vi "Omniax_mDrive_XYZ_MM_BR_RES.vi"() -> ()   [LabVIEW 2009]
uses:
  <vilib>/Instr/_visa.llb/VISA Configure Serial Port (Instr).vi
panel:
  out "Z Backlash steps/sec 2":i32
  out "Z Backlash 2":i32
  out "Z Holding Current % 2":i32
  out "Z Run Current % 2":i32
  out "Z offset mm 2":dbl
  out "Z mm/rev 2":dbl
  out "Z steps/rev 2":u32
  out "Z scan steps/sec MV step/sec 2":i32
  out "Z MINPOS 2":i32=-94296
  out "Z MAXPOS  2":i32=-34296
  out "Z COM PORT 2":refnum<visa-resource-name>="COM5"
  in  "Z Scan set 2":bool
  in  "Z Scan Velocity SP mm/sec 2":dbl
  in  "Z Scan Length SP mm 2":dbl
  in  "Z Move Set 2":bool
  out "Reset Z Motor Steps 2":i32
  in  "Reset Z Position mm 2":dbl
  out "Z Velocity MV mm/sec 2":dbl
  in  "Z Velocity SP mm/sec 2":dbl
  in  "Z Position SP mm 2":dbl
  out "Z Position MV mm 2":dbl
  out "Z Scan velocity MV mm/sec 2":dbl format="%#_6f"
  out "Z Scan length MV mm 2":dbl
  in  "Z Scan Length SP steps 2":i32 min=-460800 max=460800 step=100
  in  "Z Scan OK 2":bool
  in  "Z Velocity SP step/sec 2":i32 min=1 max=102400
  in  "Z Scan Velocity SP steps/sec 2":i32=1 min=1 max=102400 step=1
  in  "Z Go 2":bool
  in  "Z Step SP 2":i32=-20000 min=-460800 max=460800 step=500
  out "Z Position mm PV 2":dbl
  out "R Step PV":i32 max=2000
  out "Z Backlash corr 2":bool
  out "Z in Motion 2":bool
  out "Z Scan 2":bool
  out "Z in Range 2":bool
  out "Y MINPOS 3":i32=-94296
  out "Y MAXPOS 3":i32=-34296
  out "Z COM PORT":refnum<visa-resource-name>="COM5"
  out "Z Backlash steps/sec":i32
  out "Z Backlash":i32
  out "Z Holding Current %":i32
  out "Z Run Current %":i32
  out "Z offset mm":dbl
  out "Z mm/rev":dbl
  out "Z steps/rev":u32
  out "Z scan steps/sec MV step/sec":i32
  out "Z MINPOS":i32=-94296
  out "Z MAXPOS":i32=-34296
  in  "Z Scan set":bool
  in  "Z Scan Velocity SP mm/sec":dbl
  in  "Z Scan Length SP mm":dbl
  in  "Z Move Set":bool
  out "Reset Z Motor Steps":i32
  in  "Reset Z Position mm":dbl
  out "Z Velocity MV mm/sec":dbl
  in  "Z Velocity SP mm/sec":dbl
  in  "Z Position SP mm":dbl
  out "Z Position MV mm":dbl
  out "Z Scan velocity MV mm/sec":dbl format="%#_6f"
  out "Z Scan length MV mm":dbl
  in  "Z Scan Length SP steps":i32 min=-460800 max=460800 step=100
  in  "Z Scan OK":bool
  in  "Z Velocity SP step/sec":i32 min=1 max=102400
  in  "Z Scan Velocity SP steps/sec":i32=1 min=1 max=102400 step=1
  in  "Z Go":bool
  in  "Z Step SP":i32=-20000 min=-460800 max=460800 step=500
  out "Z Position mm PV":dbl
  out "Z Step PV":i32 max=2000
  out "Z Backlash corr":bool
  out "Z in Motion":bool
  out "Z Scan":bool
  out "Z in Range":bool
  out "Reset X Motor Steps":i32
  in  "Reset X Position mm":dbl
  out "X Backlash corr":bool
  out "X  in Motion":bool
  out "X Scan":bool
  out "X  in Range":bool
  out "X Step PV":i32 max=2000
  out "X Position mm PV":dbl
  out "X scan steps/sec MV step/sec":i32
  in  "X Scan set":bool
  in  "X Scan Velocity SP mm/sec":dbl
  in  "X Scan Length SP mm":dbl
  in  "X Move Set":bool
  out "X Velocity MV mm/sec":dbl
  in  "X Velocity SP mm/sec":dbl
  in  "X Position SP mm":dbl
  out "X Position MV mm":dbl
  out "X Scan velocity MV mm/sec":dbl format="%#_6f"
  out "X Scan length MV mm":dbl
  in  "X Scan Length SP steps":i32 min=-460800 max=460800 step=100
  in  "X Scan OK":bool
  in  "X Velocity SP step/sec":i32 min=1 max=102400
  in  "X Scan Velocity SP steps/sec":i32=1 min=1 max=102400 step=1
  in  "X Go":bool
  in  "X Step SP":i32=-20000 min=-460800 max=460800 step=500
  out "X Backlash steps/sec":i32
  out "X Backlash":i32
  out "X Holding Current %":i32
  out "X Run Current %":i32
  out "X offset mm":dbl
  out "X mm/rev":dbl
  out "X steps/rev":u32
  out "X MAXPOS":i32=-34296
  out "X MINPOS":i32=-94296
  out "X COM PORT":refnum<visa-resource-name>="COM5"
  out "Y Backlash corr":bool
  in  "Y Scan set":bool
  in  "Y Scan Velocity SP mm/sec":dbl
  in  "Y Scan Length SP mm":dbl
  in  "Y Move Set":bool
  out "Y Backlash steps/sec":i32
  out "Y Backlash":i32
  out "Y in Motion":bool
  in  "Reset":bool
  out "Reset Y Motor Steps":i32
  in  "Reset Y Position mm":dbl
  out "Y Velocity MV mm/sec":dbl
  in  "Y Velocity SP mm/sec":dbl
  in  "Y Position SP mm":dbl
  out "Y Position MV mm":dbl
  out "Y Holding Current %":i32
  out "Y Run Current %":i32
  out "Y Scan velocity MV mm/sec":dbl format="%#_6f"
  out "Y Scan length MV mm":dbl
  in  "Scan Cancel":bool
  out "Y Position mm PV":dbl
  out "Y offset mm":dbl
  out "Y mm/rev":dbl
  out "Y steps/rev":u32
  out "Y scan steps/sec MV step/sec":i32
  in  "Y Scan Length SP steps":i32 min=-460800 max=460800 step=100
  out "Y Scan":bool
  in  "Y Scan OK":bool
  in  "Scan Go":bool
  in  "Y Velocity SP step/sec":i32 min=1 max=102400
  in  "Y Scan Velocity SP steps/sec":i32=1 min=1 max=102400 step=1
  in  "Stop":bool
  out "Y in Range":bool
  out "Y Step PV":i32 max=2000
  in  "Y Go":bool
  in  "Y Step SP":i32=-20000 min=-460800 max=460800 step=500
  out "Y MINPOS":i32=-94296
  out "Y MAXPOS":i32=-34296
  out "Y COM PORT":refnum<visa-resource-name>="COM5"
  # "LM"
  # "MV"
  # "BL"
  # "SC"
  # "MX"
  # "MY"
  # "MZ"
  # "MR"
types:
  T1 = enum8{"Enabled", "Disabled", "Disabled and Grayed Out"}
  T2 = enum16{"Stop", "Reset", "Run Current", "Holding Current", "Accel Rate", "Decel Rate", "Move to Relative Position", "Move to Absolute Position", "Echo Mode", "Print Parameter", "Send String", "Microstep Resolution", "Set Current Position", "Max Velocity"}
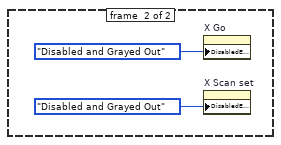
[diagram p2: hidden frame]
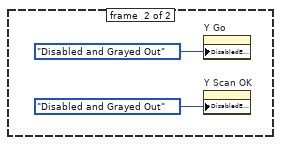
[diagram p5: hidden frame]
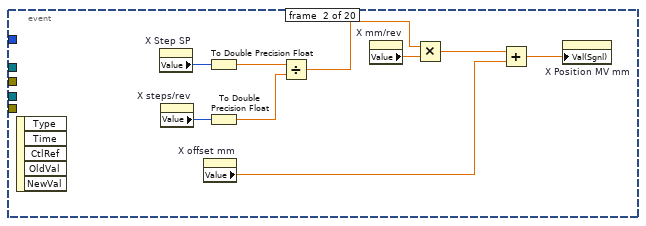
[diagram p8: hidden frame]
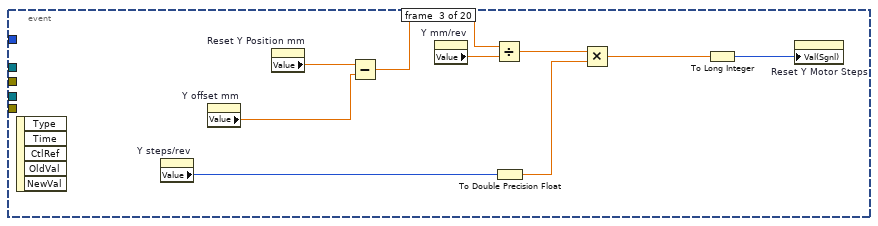
[diagram p9: hidden frame]
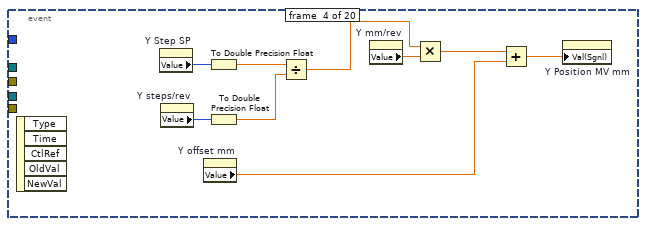
[diagram p10: hidden frame]
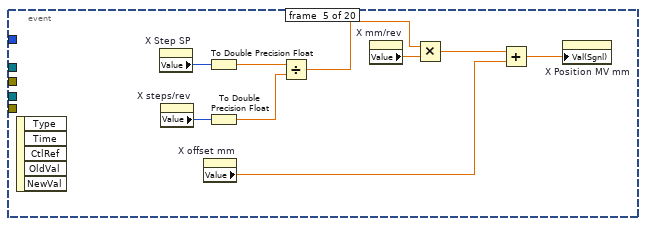
[diagram p11: hidden frame]
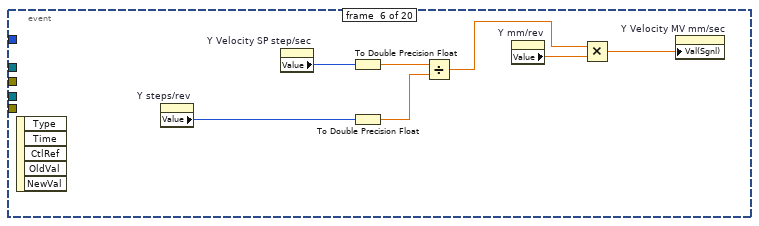
[diagram p12: hidden frame]
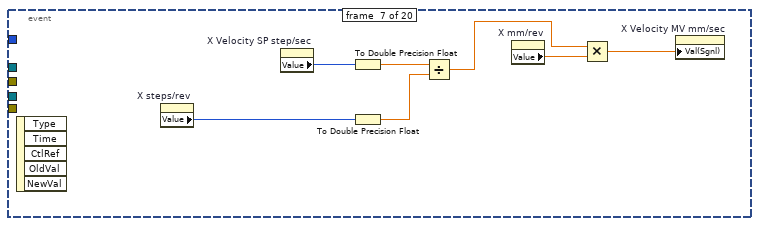
[diagram p13: hidden frame]
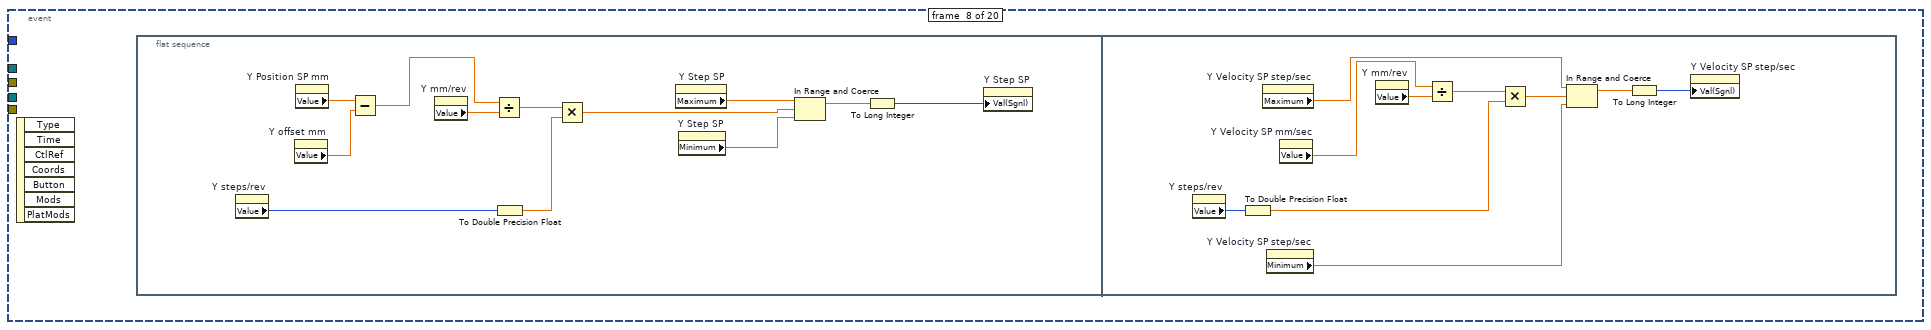
[diagram p14: hidden frame]
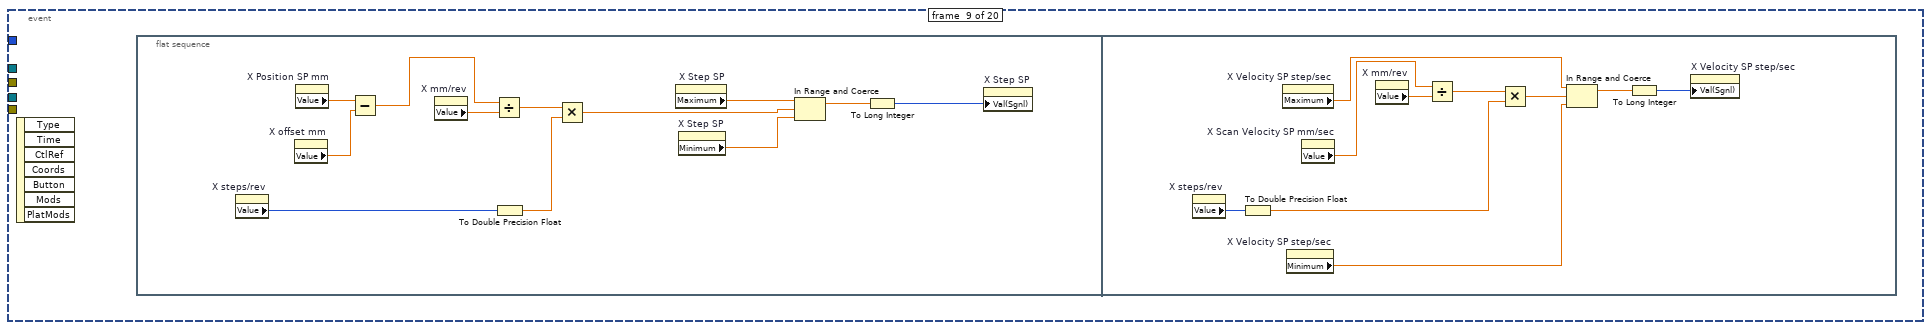
[diagram p15: hidden frame]
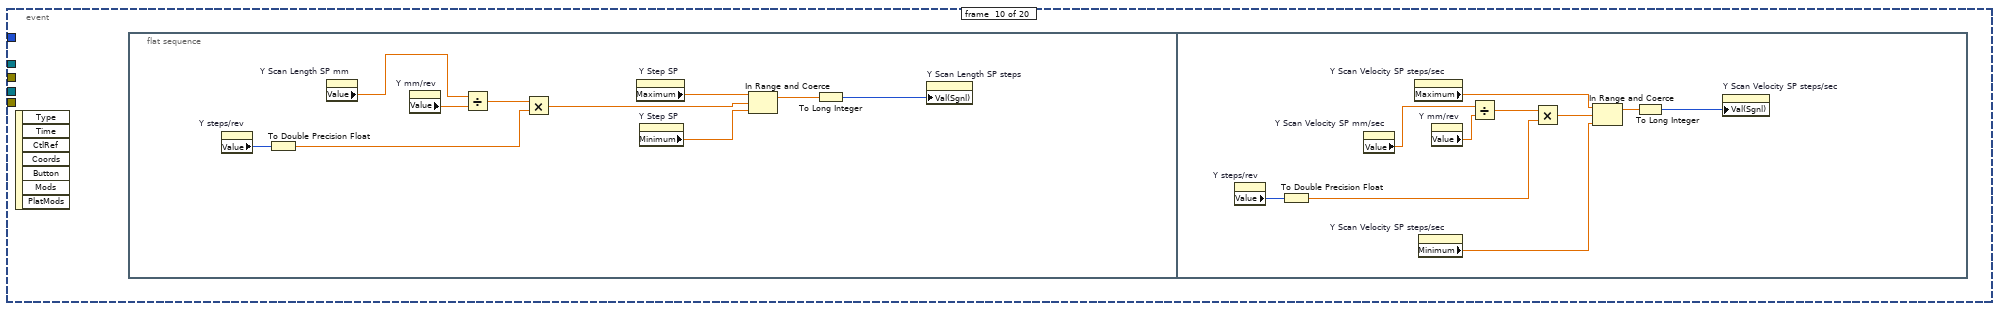
[diagram p16: hidden frame]
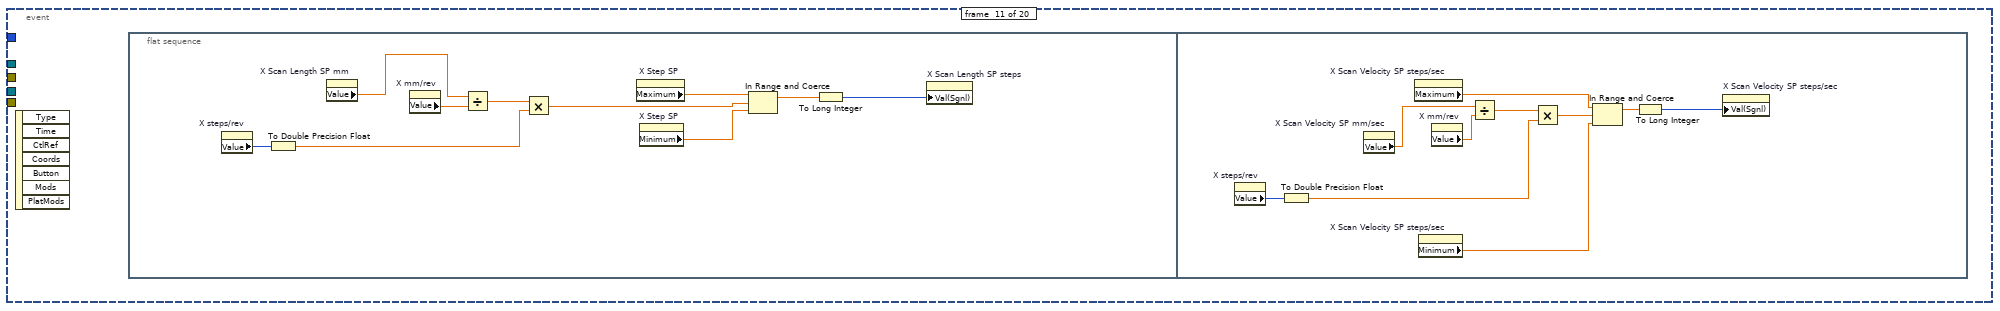
[diagram p17: hidden frame]
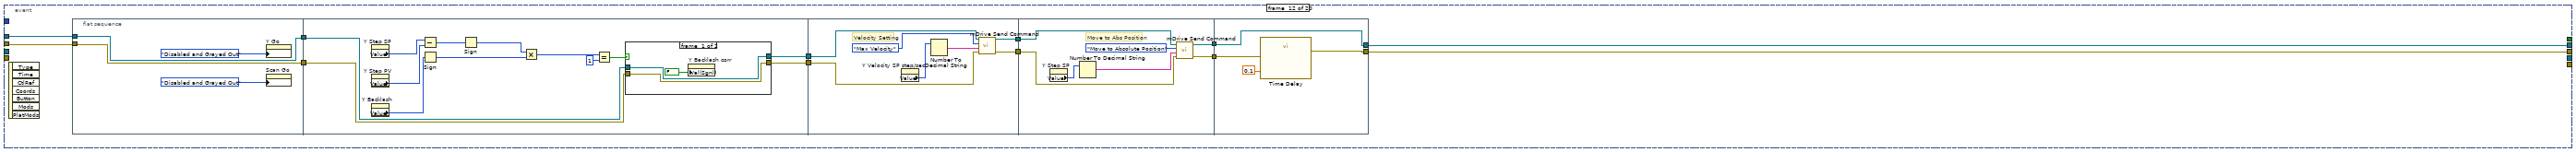
[diagram p18: hidden frame]
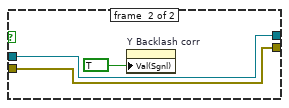
[diagram p19: hidden frame]
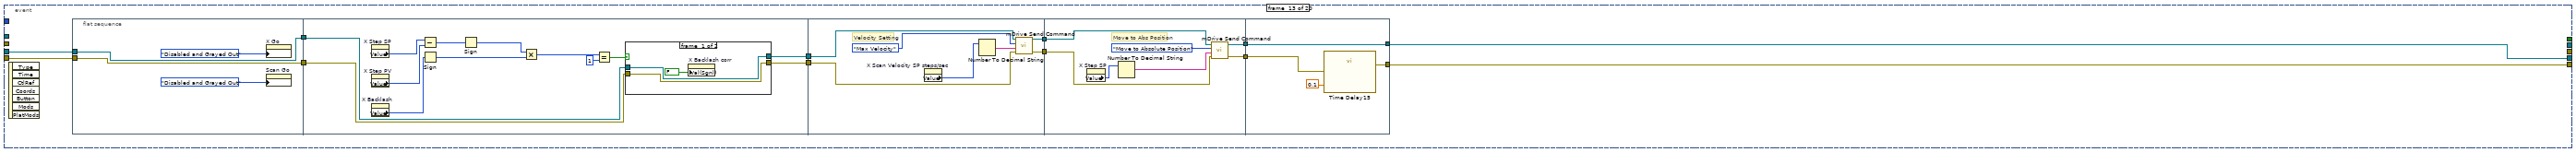
[diagram p20: hidden frame]
diagram:
  w18 = refnum<visa-resource-name> "COM10" ("COM PORT")
  w20 = u16 0 items=["None", "XON/XOFF", "RTS/CTS", "XON/XOFF & RTS/CTS", "DTR/DSR", "XON/XOFF & DTR/DSR"] ("flow control (0:none)")
  w21 = u16 10 items=["1.0"=10, "1.5"=15, "2.0"=20] ("stop bits (10: 1 bit)")
  w31 = refnum<visa-resource-name> "COM8" ("COM PORT")
  w33 = u16 0 items=["None", "XON/XOFF", "RTS/CTS", "XON/XOFF & RTS/CTS", "DTR/DSR", "XON/XOFF & DTR/DSR"] ("flow control (0:none)")
  w34 = u16 10 items=["1.0"=10, "1.5"=15, "2.0"=20] ("stop bits (10: 1 bit)")
  w58 = refnum<visa-resource-name> "COM9" ("COM PORT")
  w60 = u16 0 items=["None", "XON/XOFF", "RTS/CTS", "XON/XOFF & RTS/CTS", "DTR/DSR", "XON/XOFF & DTR/DSR"] ("flow control (0:none)")
  w61 = u16 10 items=["1.0"=10, "1.5"=15, "2.0"=20] ("stop bits (10: 1 bit)")
  # "Stop bits"
  # "Stop bits"
  # "Stop bits"
  n1 = flat-sequence {
    frame #0 {
      "Z Run Current %" <- 60 ("Z Run Current %")
      "Z Holding Current %" <- 25 ("Z Holding Current %")
    }
  }
  n2 = flat-sequence {
    frame #0 {
      w71 = 1.0 ("MM/rev")
      w74 = u32 51200 ("step/rev")
      w69 = 102400 ("Value (Signaling)")
      n3 = property on="X Backlash corr" class="Bool (strict)"("Val(Sgnl)"=FALSE ("Value (Signaling)")) -> ()  [unwired: 2 in, 2 out]
      n4 = property on="X Velocity SP step/sec" class="DigNum (strict)"("Val(Sgnl)"=w69) -> ()  [unwired: 2 in, 2 out]
      n5 = property on="X Scan Velocity SP mm/sec" class="DigNum (strict)"("Val(Sgnl)"=0.1 ("Value (Signaling)")) -> ()  [unwired: 2 in, 2 out]
      n6 = property on="X Scan" class="Bool (strict)"("Val(Sgnl)"=FALSE ("Value (Signaling)")) -> ()  [unwired: 2 in, 2 out]
      n7 = property on="X Velocity SP step/sec" class="DigNum (strict)"("Minimum"=1.0 ("Data Entry Limits:Minimum")) -> ()  [unwired: 2 in, 2 out]
      n8 = To Double Precision Float(number=w74) -> (double precision float=w73:dbl)
      n9 = To Double Precision Float(number=w69) -> (double precision float=w75:dbl)
      n10 = Divide(x=w75, y=w73) -> (x/y=w70:dbl)
      n11 = property on="X Velocity SP step/sec" class="DigNum (strict)"("Maximum"=w75) -> ()  [unwired: 2 in, 2 out]
      n12 = Multiply(x=w70, y=w71) -> (x*y=w72:dbl)
      n13 = property on="X Velocity SP mm/sec" class="DigNum (strict)"("Val(Sgnl)"=w72) -> ()  [unwired: 2 in, 2 out]
      "X Run Current %" <- 60 ("Run Current %")
      "X Holding Current %" <- 25 ("Holding Current %")
      "X Backlash" <- -5120 ("Backlash2")
      "X Backlash steps/sec" <- 25600 ("Value (Signaling)")
      "X offset mm" <- 0.0 ("offset")
      "X steps/rev" <- w74
      "X mm/rev" <- w71
    }
  }
  n14 = flat-sequence {
    frame #0 {
      w87 = 1.0 ("MM/rev")
      w90 = u32 51200 ("step/rev")
      w85 = 102400 ("Value (Signaling)")
      n15 = property on="Y Backlash corr" class="Bool (strict)"("Val(Sgnl)"=FALSE ("Value (Signaling)")) -> ()  [unwired: 2 in, 2 out]
      n16 = property on="Y Velocity SP step/sec" class="DigNum (strict)"("Val(Sgnl)"=w85) -> ()  [unwired: 2 in, 2 out]
      n17 = property on="Y Scan Velocity SP mm/sec" class="DigNum (strict)"("Val(Sgnl)"=0.1 ("Value (Signaling)")) -> ()  [unwired: 2 in, 2 out]
      n18 = property on="Y Scan" class="Bool (strict)"("Val(Sgnl)"=FALSE ("Value (Signaling)")) -> ()  [unwired: 2 in, 2 out]
      n19 = property on="Y Velocity SP step/sec" class="DigNum (strict)"("Minimum"=1.0 ("Data Entry Limits:Minimum")) -> ()  [unwired: 2 in, 2 out]
      n20 = To Double Precision Float(number=w90) -> (double precision float=w89:dbl)
      n21 = To Double Precision Float(number=w85) -> (double precision float=w91:dbl)
      n22 = Divide(x=w91, y=w89) -> (x/y=w86:dbl)
      n23 = property on="Y Velocity SP step/sec" class="DigNum (strict)"("Maximum"=w91) -> ()  [unwired: 2 in, 2 out]
      n24 = Multiply(x=w86, y=w87) -> (x*y=w88:dbl)
      n25 = property on="Y Velocity SP mm/sec" class="DigNum (strict)"("Val(Sgnl)"=w88) -> ()  [unwired: 2 in, 2 out]
      "Y Backlash" <- -5120 ("Backlash2")
      "Y Backlash steps/sec" <- 25600 ("Value (Signaling)")
      "Y Run Current %" <- 60 ("Run Current %")
      "Y Holding Current %" <- 25 ("Holding Current %")
      "Y offset mm" <- 0.0 ("offset")
      "Y steps/rev" <- w90
      "Y mm/rev" <- w87
    }
  }
  n26 = property on="Scan Go" class="Bool"("DisabledEnum"=T1."Disabled and Grayed Out" ("Disabled")) -> ()  [unwired: 2 in, 2 out]
  n27 = property on="Scan Cancel" class="Bool"("DisabledEnum"=T1."Disabled and Grayed Out" ("Disabled")) -> ()  [unwired: 2 in, 2 out]
  n28 = call-poly "VISA Configure Serial Port"("VISA resource name"=w58, "timeout (10sec)"=u32 10000, "baud rate (9600)"=u32 9600, "data bits (8)"=u16 8, "parity (0:none)"=enum16{"None", "Odd", "Even", "Mark", "Space"}."None", "stop bits (10: 1 bit)"=w61, "flow control (0:none)"=w60) -> ("VISA resource name out"=w51:refnum<visa-resource-name>, "error out"=w50:errorcluster)  [unwired: 7 in]
  n29 = call-poly "VISA Configure Serial Port"("VISA resource name"=w31, "timeout (10sec)"=u32 10000, "baud rate (9600)"=u32 9600, "data bits (8)"=u16 8, "parity (0:none)"=enum16{"None", "Odd", "Even", "Mark", "Space"}."None", "stop bits (10: 1 bit)"=w34, "flow control (0:none)"=w33) -> ("VISA resource name out"=w30:refnum<visa-resource-name>, "error out"=w29:errorcluster)  [unwired: 7 in]
  n30 = call-poly "VISA Configure Serial Port"("VISA resource name"=w18, "timeout (10sec)"=u32 10000, "baud rate (9600)"=u32 9600, "data bits (8)"=u16 8, "parity (0:none)"=enum16{"None", "Odd", "Even", "Mark", "Space"}."None", "stop bits (10: 1 bit)"=w21, "flow control (0:none)"=w20) -> ("VISA resource name out"=w2:refnum<visa-resource-name>, "error out"=w1:errorcluster)  [unwired: 7 in]
  n31 = flat-sequence {
    tunnel: w50 -> [w105]
    tunnel: w51 -> [w103]
    tunnel: [w102] -> w47
    tunnel: [w104] -> w45
    tunnel: w47 -> [w112]
    tunnel: [w111] -> w46
    tunnel: w45 -> [w109]
    tunnel: [w110] -> w44
    tunnel: [w122] -> w53
    tunnel: [w123] -> w52
    tunnel: w46 -> [w121]
    tunnel: w44 -> [w120]
    tunnel: w53 -> [w133]
    tunnel: w52 -> [w132]
    tunnel: [w135] -> w17
    tunnel: [w134] -> w16
    tunnel: [w129] -> w15
    tunnel: [w140] -> w56
    tunnel: [w141] -> w57
    tunnel: w17 -> [w141]
    tunnel: w16 -> [w140]
    tunnel: w15 -> [w136]
    frame #0 {
      # "Run Current %"
      n32 = property on="Y Run Current %" class="DigNum (strict)"() -> ("Value"=w100:i32)  [unwired: 2 in, 2 out]
      n33 = Number To Decimal String(number=w100) -> (decimal integer string=w101:string)  [unwired: 1 in]
      n34 = call "mDrive Send Command.vi"("error in (no error)"=w105, "Extra"=w101, "Command"=T2."Run Current", "VISA resource name"=w103) -> ("error out"=w104:errorcluster, "VISA resource name out"=w102:refnum<visa-resource-name>)  [unwired: 3 in, 1 out]
    }
    frame #1 {
      # "Holding Current %"
      n35 = property on="Y Holding Current %" class="DigNum (strict)"() -> ("Value"=w107:i32)  [unwired: 2 in, 2 out]
      n36 = Number To Decimal String(number=w107) -> (decimal integer string=w108:string)  [unwired: 1 in]
      n37 = call "mDrive Send Command.vi"("error in (no error)"=w109, "Extra"=w108, "Command"=T2."Holding Current", "VISA resource name"=w112) -> ("error out"=w110:errorcluster, "VISA resource name out"=w111:refnum<visa-resource-name>)  [unwired: 3 in, 1 out]
    }
    frame #2 {
      # "Print Velocity Ma"
      # "Velocity Max"
      n38 = property on="Y Velocity SP step/sec" class="DigNum (strict)"() -> ("Value"=w119:i32)  [unwired: 2 in, 2 out]
      n39 = Number To Decimal String(number=w119) -> (decimal integer string=w118:string)  [unwired: 1 in]
      n40 = call "mDrive Send Command.vi"("error in (no error)"=w120, "Extra"=w118, "Command"=T2."Max Velocity", "VISA resource name"=w121) -> ("error out"=w116:errorcluster, "VISA resource name out"=w126:refnum<visa-resource-name>)  [unwired: 3 in, 1 out]
      n41 = call "mDrive Send Command.vi"("error in (no error)"=w116, "Extra"="VM", "Command"=T2."Print Parameter", "VISA resource name"=w126) -> ("error out"=w123:errorcluster, "read buffer"=w124:string, "VISA resource name out"=w122:refnum<visa-resource-name>)  [unwired: 3 in]
      n42 = Decimal String To Number(string=w124, offset=0) -> (number=w117:i32)  [unwired: 1 in, 1 out]
      n43 = property on="Y scan steps/sec MV step/sec" class="DigNum (strict)"("Val(Sgnl)"=w117) -> ()  [unwired: 2 in, 2 out]
    }
    frame #3 {
      # "PRINT POSITION"
      n44 = call "mDrive Send Command.vi"("error in (no error)"=w132, "Extra"="P", "Command"=T2."Print Parameter", "VISA resource name"=w133) -> ("error out"=w134:errorcluster, "read buffer"=w131:string, "VISA resource name out"=w135:refnum<visa-resource-name>)  [unwired: 3 in]
      n45 = Decimal String To Number(string=w131, offset=0) -> (number=w129:i32)  [unwired: 1 in, 1 out]
    }
    frame #4 {
      w138 = -460800 ("lower limit")
      w139 = 460800 ("upper limit")
      n46 = property on="Y Step SP" class="DigNum (strict)"("Val(Sgnl)"=w136) -> ()  [unwired: 2 in, 2 out]
      n47 = property on="Y Step SP" class="DigNum (strict)"("Maximum"=w139) -> ()  [unwired: 2 in, 2 out]
      n48 = property on="Y Step SP" class="DigNum (strict)"("Minimum"=w138) -> ()  [unwired: 2 in, 2 out]
      n49 = In Range and Coerce(upper limit=w139, x=w136, lower limit=w138) -> (In Range?=w137:bool)  [unwired: 1 out]
      n50 = property on="Y in Range" class="Bool (strict)"("Val(Sgnl)"=w137) -> ()  [unwired: 2 in, 2 out]
      "Y MINPOS" <- w138
      "Y MAXPOS" <- w139
    }
  }
  n51 = flat-sequence {
    tunnel: w29 -> [w148]
    tunnel: w30 -> [w146]
    tunnel: [w145] -> w43
    tunnel: [w147] -> w42
    tunnel: w43 -> [w155]
    tunnel: [w154] -> w41
    tunnel: w42 -> [w152]
    tunnel: [w153] -> w40
    tunnel: [w165] -> w39
    tunnel: [w166] -> w38
    tunnel: w41 -> [w164]
    tunnel: w40 -> [w163]
    tunnel: w39 -> [w176]
    tunnel: w38 -> [w175]
    tunnel: [w178] -> w14
    tunnel: [w177] -> w13
    tunnel: [w172] -> w12
    tunnel: [w183] -> w27
    tunnel: [w184] -> w28
    tunnel: w14 -> [w184]
    tunnel: w13 -> [w183]
    tunnel: w12 -> [w179]
    frame #0 {
      # "Run Current %"
      n52 = property on="X Run Current %" class="DigNum (strict)"() -> ("Value"=w143:i32)  [unwired: 2 in, 2 out]
      n53 = Number To Decimal String(number=w143) -> (decimal integer string=w144:string)  [unwired: 1 in]
      n54 = call "mDrive Send Command.vi"("error in (no error)"=w148, "Extra"=w144, "Command"=T2."Run Current", "VISA resource name"=w146) -> ("error out"=w147:errorcluster, "VISA resource name out"=w145:refnum<visa-resource-name>)  [unwired: 3 in, 1 out]
    }
    frame #1 {
      # "Holding Current %"
      n55 = property on="X Holding Current %" class="DigNum (strict)"() -> ("Value"=w150:i32)  [unwired: 2 in, 2 out]
      n56 = Number To Decimal String(number=w150) -> (decimal integer string=w151:string)  [unwired: 1 in]
      n57 = call "mDrive Send Command.vi"("error in (no error)"=w152, "Extra"=w151, "Command"=T2."Holding Current", "VISA resource name"=w155) -> ("error out"=w153:errorcluster, "VISA resource name out"=w154:refnum<visa-resource-name>)  [unwired: 3 in, 1 out]
    }
    frame #2 {
      # "Print Velocity Ma"
      # "Velocity Max"
      n58 = property on="X Velocity SP step/sec" class="DigNum (strict)"() -> ("Value"=w162:i32)  [unwired: 2 in, 2 out]
      n59 = Number To Decimal String(number=w162) -> (decimal integer string=w161:string)  [unwired: 1 in]
      n60 = call "mDrive Send Command.vi"("error in (no error)"=w163, "Extra"=w161, "Command"=T2."Max Velocity", "VISA resource name"=w164) -> ("error out"=w159:errorcluster, "VISA resource name out"=w169:refnum<visa-resource-name>)  [unwired: 3 in, 1 out]
      n61 = call "mDrive Send Command.vi"("error in (no error)"=w159, "Extra"="VM", "Command"=T2."Print Parameter", "VISA resource name"=w169) -> ("error out"=w166:errorcluster, "read buffer"=w167:string, "VISA resource name out"=w165:refnum<visa-resource-name>)  [unwired: 3 in]
      n62 = Decimal String To Number(string=w167, offset=0) -> (number=w160:i32)  [unwired: 1 in, 1 out]
      n63 = property on="X scan steps/sec MV step/sec" class="DigNum (strict)"("Val(Sgnl)"=w160) -> ()  [unwired: 2 in, 2 out]
    }
    frame #3 {
      # "PRINT POSITION"
      n64 = call "mDrive Send Command.vi"("error in (no error)"=w175, "Extra"="P", "Command"=T2."Print Parameter", "VISA resource name"=w176) -> ("error out"=w177:errorcluster, "read buffer"=w174:string, "VISA resource name out"=w178:refnum<visa-resource-name>)  [unwired: 3 in]
      n65 = Decimal String To Number(string=w174, offset=0) -> (number=w172:i32)  [unwired: 1 in, 1 out]
    }
    frame #4 {
      w181 = -460800 ("lower limit")
      w182 = 460800 ("upper limit")
      n66 = property on="X Step SP" class="DigNum (strict)"("Val(Sgnl)"=w179) -> ()  [unwired: 2 in, 2 out]
      n67 = property on="X Step SP" class="DigNum (strict)"("Maximum"=w182) -> ()  [unwired: 2 in, 2 out]
      n68 = property on="X Step SP" class="DigNum (strict)"("Minimum"=w181) -> ()  [unwired: 2 in, 2 out]
      n69 = In Range and Coerce(upper limit=w182, x=w179, lower limit=w181) -> (In Range?=w180:bool)  [unwired: 1 out]
      n70 = property on="X  in Range" class="Bool (strict)"("Val(Sgnl)"=w180) -> ()  [unwired: 2 in, 2 out]
      "X MINPOS" <- w181
      "X MAXPOS" <- w182
    }
  }
  n71 = flat-sequence {
    tunnel: w1 -> [w191]
    tunnel: w2 -> [w189]
    tunnel: [w188] -> w11
    tunnel: [w190] -> w10
    tunnel: w11 -> [w198]
    tunnel: [w197] -> w9
    tunnel: w10 -> [w195]
    tunnel: [w196] -> w8
    tunnel: [w208] -> w7
    tunnel: [w209] -> w6
    tunnel: w9 -> [w207]
    tunnel: w8 -> [w206]
    tunnel: w7 -> [w219]
    tunnel: w6 -> [w218]
    tunnel: [w221] -> w5
    tunnel: [w220] -> w4
    tunnel: [w215] -> w3
    tunnel: [w226] -> _
    tunnel: [w227] -> _
    tunnel: w5 -> [w227]
    tunnel: w4 -> [w226]
    tunnel: w3 -> [w222]
    frame #0 {
      # "Run Current %"
      n72 = property on="Property Node" class="DigNum (strict)"() -> ("Value"=w186:i32)  [unwired: 2 in, 2 out]
      n73 = Number To Decimal String(number=w186) -> (decimal integer string=w187:string)  [unwired: 1 in]
      n74 = call "mDrive Send Command.vi"("error in (no error)"=w191, "Extra"=w187, "Command"=T2."Run Current", "VISA resource name"=w189) -> ("error out"=w190:errorcluster, "VISA resource name out"=w188:refnum<visa-resource-name>)  [unwired: 3 in, 1 out]
    }
    frame #1 {
      # "Holding Current %"
      n75 = property on="Property Node" class="DigNum (strict)"() -> ("Value"=w193:i32)  [unwired: 2 in, 2 out]
      n76 = Number To Decimal String(number=w193) -> (decimal integer string=w194:string)  [unwired: 1 in]
      n77 = call "mDrive Send Command.vi"("error in (no error)"=w195, "Extra"=w194, "Command"=T2."Holding Current", "VISA resource name"=w198) -> ("error out"=w196:errorcluster, "VISA resource name out"=w197:refnum<visa-resource-name>)  [unwired: 3 in, 1 out]
    }
    frame #2 {
      # "Print Velocity Ma"
      # "Velocity Max"
      n78 = property on="Property Node" class="DigNum (strict)"() -> ("Value"=w205:i32)  [unwired: 2 in, 2 out]
      n79 = Number To Decimal String(number=w205) -> (decimal integer string=w204:string)  [unwired: 1 in]
      n80 = call "mDrive Send Command.vi"("error in (no error)"=w206, "Extra"=w204, "Command"=T2."Max Velocity", "VISA resource name"=w207) -> ("error out"=w202:errorcluster, "VISA resource name out"=w212:refnum<visa-resource-name>)  [unwired: 3 in, 1 out]
      n81 = call "mDrive Send Command.vi"("error in (no error)"=w202, "Extra"="VM", "Command"=T2."Print Parameter", "VISA resource name"=w212) -> ("error out"=w209:errorcluster, "read buffer"=w210:string, "VISA resource name out"=w208:refnum<visa-resource-name>)  [unwired: 3 in]
      n82 = Decimal String To Number(string=w210, offset=0) -> (number=w203:i32)  [unwired: 1 in, 1 out]
      n83 = property on="Property Node" class="DigNum (strict)"("Val(Sgnl)"=w203) -> ()  [unwired: 2 in, 2 out]
    }
    frame #3 {
      # "PRINT POSITION"
      n84 = call "mDrive Send Command.vi"("error in (no error)"=w218, "Extra"="P", "Command"=T2."Print Parameter", "VISA resource name"=w219) -> ("error out"=w220:errorcluster, "read buffer"=w217:string, "VISA resource name out"=w221:refnum<visa-resource-name>)  [unwired: 3 in]
      n85 = Decimal String To Number(string=w217, offset=0) -> (number=w215:i32)  [unwired: 1 in, 1 out]
    }
    frame #4 {
      w224 = -460800 ("lower limit")
      w225 = 460800 ("upper limit")
      n86 = property on="Property Node" class="DigNum (strict)"("Val(Sgnl)"=w222) -> ()  [unwired: 2 in, 2 out]
      n87 = property on="Property Node" class="DigNum (strict)"("Maximum"=w225) -> ()  [unwired: 2 in, 2 out]
      n88 = In Range and Coerce(upper limit=w225, x=w222, lower limit=w224) -> (In Range?=w223:bool)  [unwired: 1 out]
      n89 = property on="Property Node" class="DigNum (strict)"("Minimum"=w224) -> ()  [unwired: 2 in, 2 out]
      n90 = property on="Property Node" class="Bool (strict)"("Val(Sgnl)"=w223) -> ()  [unwired: 2 in, 2 out]
      "Y MINPOS 3" <- w224
      "Y MAXPOS 3" <- w225
    }
  }
  n91 = while {
    tunnel: w57 -> [w234]
    tunnel: w56 -> [w237]
    tunnel: [w238] -> w54
    tunnel: [w236] -> w55
    tunnel: w28 -> [w231]
    tunnel: w27 -> [w230]
    tunnel: [w229] -> w26
    tunnel: [w228] -> w25
    stop <- w233 stop-if-true
    n92 = flat-sequence {
      frame #0 {
      }
    }
    n93 = flat-sequence {
      frame #0 {
      }
    }
    n94 = property on="Y steps/rev" class="DigNum (strict)"() -> ("Value"=w232:u32)  [unwired: 2 in, 2 out]
    n95 = event shown="[18] \"Scan Go\": Mouse Up" {
      selector: _ -> [_ _ _ _ _ _ _ _ _ _ _ _ _ _ _ _ _ _ _ _]
      dyn-events: _ -> [_ _ _ _ _ _ _ _ _ _ _ _ _ _ _ _ _ _ _ _]
      timeout: 500 -> [_ _ _ _ _ _ _ _ _ _ _ _ _ _ _ _ _ _ _ _]
      tunnel: w237 -> [w272 _ _ _ _ _ _ _ _ _ _ w707 _ _ w851 w880 w890 w902 w948 w1004]
      tunnel: [w271 _ _ _ _ _ _ _ _ _ _ w713 _ _ w849 w880 w888 w904 w945 w1002] -> w238
      tunnel: w234 -> [w269 _ _ _ _ _ _ _ _ _ _ w708 _ _ w850 w881 w891 w903 w947 w1005]
      tunnel: [w270 _ _ _ _ _ _ _ _ _ _ w714 _ _ w846 w881 w889 w905 w946 w1003] -> w236
      tunnel: [_ _ _ _ _ _ _ _ _ _ _ _ _ _ _ TRUE _ _ _ _] -> w233
      tunnel: w232 -> [_ _ _ _ _ _ _ _ _ _ _ _ _ _ _ _ _ _ _ _]
      tunnel: w231 -> [w242 _ _ _ _ _ _ _ _ _ _ _ w759 w814 _ _ w883 w895 _ w1001]
      tunnel: w230 -> [w241 _ _ _ _ _ _ _ _ _ _ _ w758 w813 _ _ w882 w894 _ w1000]
      tunnel: [w240 _ _ _ _ _ _ _ _ _ _ _ w757 w812 _ _ w885 w893 _ w999] -> w229
      tunnel: [w239 _ _ _ _ _ _ _ _ _ _ _ w756 w811 _ _ w884 w892 _ w998] -> w228
      event #0 {
        n96 = event-data() -> ()  [unwired: 1 in, 2 out]
        n97 = flat-sequence {
          tunnel: w272 -> [w451]
          tunnel: w269 -> [w450]
          tunnel: [w456] -> w268
          tunnel: [w430] -> w266
          tunnel: [w443] -> w264
          tunnel: [w421] -> w262
          tunnel: w268 -> [w462]
          tunnel: [w462] -> w267
          tunnel: w266 -> [w461]
          tunnel: [w461] -> w265
          tunnel: w264 -> [w460]
          tunnel: [w460] -> w263
          tunnel: w262 -> [w457]
          tunnel: [w457] -> w257
          tunnel: w267 -> [w469]
          tunnel: [w470] -> w261
          tunnel: w265 -> [w472]
          tunnel: [w471] -> w260
          tunnel: w263 -> [w468]
          tunnel: [w467] -> w258
          tunnel: w257 -> [w467]
          tunnel: w261 -> [w482]
          tunnel: w260 -> [w483]
          tunnel: [w481] -> w259
          tunnel: w258 -> [w485]
          tunnel: [w480] -> w256
          tunnel: [w567] -> w271
          tunnel: [w568] -> w270
          tunnel: w259 -> [w567]
          tunnel: w256 -> [w568]
          frame #0 {
            w425 = 0.1 ("Delay Time (s)")
            n98 = property on="Y Step SP" class="DigNum (strict)"() -> ("Maximum"=w445:dbl)  [unwired: 2 in, 2 out]
            n99 = property on="Y Step SP" class="DigNum (strict)"() -> ("Minimum"=w447:dbl)  [unwired: 2 in, 2 out]
            n100 = property on="Y steps/rev" class="DigNum (strict)"() -> ("Value"=w441:u32)  [unwired: 2 in, 2 out]
            n101 = property on="Y offset mm" class="DigNum (strict)"() -> ("Value"=w437:dbl)  [unwired: 2 in, 2 out]
            n102 = call "mDrive Send Command.vi"("error in (no error)"=w451, "Extra"="P", "Command"=T2."Print Parameter", "VISA resource name"=w450) -> ("error out"=w449:errorcluster, "read buffer"=w455:string, "VISA resource name out"=w453:refnum<visa-resource-name>)  [unwired: 3 in]
            n103 = call "Time Delay4"("error in (no error)"=w449, "Delay Time (s)"=w425) -> ("error out"=w448:errorcluster)  [unwired: 9 in]
            n104 = Decimal String To Number(string=w455, offset=0) -> (number=w433:i32)  [unwired: 1 in, 1 out]
            n105 = To Long Integer(number=w433) -> (32bit integer=w435:i32)
            n106 = property on="Y Step PV" class="DigNum (strict)"("Val(Sgnl)"=w435) -> ()  [unwired: 2 in, 2 out]
            n107 = To Long Integer(number=w445) -> (32bit integer=w444:i32)
            n108 = To Long Integer(number=w447) -> (32bit integer=w446:i32)
            n109 = call "mDrive Send Command.vi"("error in (no error)"=w448, "Extra"="MV", "Command"=T2."Print Parameter", "VISA resource name"=w453) -> ("error out"=w452:errorcluster, "read buffer"=w431:string, "VISA resource name out"=w456:refnum<visa-resource-name>)  [unwired: 3 in]
            n110 = call "Time Delay3"("error in (no error)"=w452, "Delay Time (s)"=w425) -> ("error out"=w430:errorcluster)  [unwired: 9 in]
            n111 = In Range and Coerce(upper limit=w444, x=w435, lower limit=w446) -> (In Range?=w443:bool)  [unwired: 1 out]
            n112 = To Double Precision Float(number=w435) -> (double precision float=w436:dbl)
            n113 = To Double Precision Float(number=w441) -> (double precision float=w442:dbl)
            n114 = Decimal String To Number(string=w431, offset=0 ("offset (0)")) -> (number=w424:i32)  [unwired: 1 in, 1 out]
            n115 = property on="Y in Range" class="Bool (strict)"("Val(Sgnl)"=w443) -> ()  [unwired: 2 in, 2 out]
            n116 = Divide(x=w436, y=w442) -> (x/y=w440:dbl)
            n117 = Number To Boolean Array(number=w424) -> (Boolean array=w423:bool[])
            n118 = property on="Y mm/rev" class="DigNum (strict)"() -> ("Value"=w439:dbl)  [unwired: 2 in, 2 out]
            n119 = Index Array(array=w423, index=0) -> (element=w421:bool)
            n120 = property on="Y in Motion" class="Bool (strict)"("Val(Sgnl)"=w421) -> ()  [unwired: 2 in, 2 out]
            n121 = Multiply(x=w440, y=w439) -> (x*y=w438:dbl)
            n122 = Add(x=w438, y=w437) -> (x+y=w434:dbl)
            n123 = property on="Y Position mm PV" class="DigNum (strict)"("Val(Sgnl)"=w434) -> ()  [unwired: 2 in, 2 out]
          }
          frame #1 {
            n124 = property on="Y Scan" class="Bool (strict)"() -> ("Value"=w458:bool)  [unwired: 2 in, 2 out]
            n125 = Or(x=w457, y=w458) -> (x .or. y?=w459:bool)
            n126 = case shown="False" w459 {
              frame #0 {
                n127 = property on="Y Go" class="Bool"("DisabledEnum"=T1."Enabled" ("Disabled")) -> ()  [unwired: 2 in, 2 out]
                n128 = property on="Y Scan OK" class="Bool"("DisabledEnum"=T1."Enabled" ("Disabled")) -> ()  [unwired: 2 in, 2 out]
              }
              frame #1 {
                n129 = property on="Y Go" class="Bool"("DisabledEnum"=T1."Disabled and Grayed Out" ("Disabled")) -> ()  [unwired: 2 in, 2 out]
                n130 = property on="Y Scan OK" class="Bool"("DisabledEnum"=T1."Disabled and Grayed Out" ("Disabled")) -> ()  [unwired: 2 in, 2 out]
              }
            }
          }
          frame #2 {
            n131 = case shown="False" w468 {
              tunnel: w469 -> [w475 w479]
              tunnel: [w476 w479] -> w470
              tunnel: [w477 w478] -> w471
              tunnel: w472 -> [w474 w478]
              frame #0 {
                n132 = call "mDrive Send Command.vi"("error in (no error)"=w474, "Command"=T2."Stop", "VISA resource name"=w475) -> ("error out"=w477:errorcluster, "VISA resource name out"=w476:refnum<visa-resource-name>)  [unwired: 4 in, 1 out]
              }
              frame #1 {
              }
            }
          }
          frame #3 {
            n133 = property on="Y Backlash corr" class="Bool (strict)"() -> ("Value"=w486:bool)  [unwired: 2 in, 2 out]
            n134 = Implies(1:w485, 2:w486) -> (0:w484:bool)
            n135 = case shown="False" w484 {
              tunnel: w483 -> [w493 w546]
              tunnel: w482 -> [w492 w547]
              tunnel: [w491 w546] -> w481
              tunnel: [w490 w547] -> w480
              frame #0 {
                # "Backlash"
                n136 = flat-sequence {
                  tunnel: [w508] -> w505
                  tunnel: [w510] -> w504
                  tunnel: [w509] -> w503
                  tunnel: w493 -> [w507]
                  tunnel: w492 -> [w506]
                  tunnel: w505 -> [w518]
                  tunnel: [w518] -> w502
                  tunnel: w504 -> [w517]
                  tunnel: w503 -> [w516]
                  tunnel: [w515] -> w501
                  tunnel: [w514] -> w500
                  tunnel: [w513] -> w489
                  tunnel: w502 -> [w528]
                  tunnel: w501 -> [w527]
                  tunnel: w500 -> [w525]
                  tunnel: [w526] -> w499
                  tunnel: [w525] -> w498
                  tunnel: [w524] -> w495
                  tunnel: [w523] -> w494
                  tunnel: w489 -> [w523]
                  tunnel: w499 -> [w539]
                  tunnel: w498 -> [w532]
                  tunnel: [w539] -> w497
                  tunnel: [w538] -> w496
                  tunnel: w495 -> [w538]
                  tunnel: w494 -> [w534]
                  tunnel: [w533] -> w487
                  tunnel: w497 -> [w543]
                  tunnel: w496 -> [w542]
                  tunnel: [w541] -> w491
                  tunnel: [w540] -> w488
                  tunnel: w487 -> [w540]
                  tunnel: [w545] -> w490
                  tunnel: w488 -> [w545]
                  frame #0 {
                    n137 = property on="Y Backlash steps/sec" class="DigNum (strict)"() -> ("Value"=w508:i32)  [unwired: 2 in, 2 out]
                    n138 = Number To Decimal String(number=w508) -> (decimal integer string=w511:string)  [unwired: 1 in]
                    n139 = call "mDrive Send Command.vi"("error in (no error)"=w507, "Extra"=w511, "Command"=T2."Max Velocity", "VISA resource name"=w506) -> ("error out"=w509:errorcluster, "VISA resource name out"=w510:refnum<visa-resource-name>)  [unwired: 3 in, 1 out]
                  }
                  frame #1 {
                    n140 = property on="Y Backlash" class="DigNum (strict)"() -> ("Value"=w513:i32)  [unwired: 2 in, 2 out]
                    n141 = Number To Decimal String(number=w513) -> (decimal integer string=w519:string)  [unwired: 1 in]
                    n142 = call "mDrive Send Command.vi"("error in (no error)"=w516, "Extra"=w519, "Command"=T2."Move to Relative Position", "VISA resource name"=w517) -> ("error out"=w515:errorcluster, "VISA resource name out"=w514:refnum<visa-resource-name>)  [unwired: 3 in, 1 out]
                  }
                  frame #2 {
                    n143 = To Double Precision Float(number=w523) -> (double precision float=w521:dbl)
                    n144 = To Double Precision Float(number=w528) -> (double precision float=w530:dbl)
                    n145 = Absolute Value(x=w521) -> (abs(x)=w522:dbl)
                    n146 = Divide(x=w522, y=w530) -> (x/y=w531:dbl)
                    n147 = Add(x=w531, y=0.3) -> (x+y=w524:dbl)
                    n148 = call "Time Delay8"("error in (no error)"=w527, "Delay Time (s)"=w524) -> ("error out"=w526:errorcluster)  [unwired: 9 in]
                  }
                  frame #3 {
                    n149 = Negate(x=w534) -> (-x=w535:i32)
                    n150 = Number To Decimal String(number=w535) -> (decimal integer string=w536:string)  [unwired: 1 in]
                    n151 = call "mDrive Send Command.vi"("Extra"=w536, "Command"=T2."Move to Relative Position", "VISA resource name"=w532) -> ("VISA resource name out"=w533:refnum<visa-resource-name>)  [unwired: 4 in, 2 out]
                  }
                  frame #4 {
                    n152 = call "Time Delay2"("error in (no error)"=w543, "Delay Time (s)"=w542) -> ("error out"=w541:errorcluster)  [unwired: 9 in]
                  }
                  frame #5 {
                    n153 = property on="Y Backlash corr" class="Bool (strict)"("Val(Sgnl)"=FALSE ("Value (Signaling)")) -> ()  [unwired: 2 in, 2 out]
                  }
                }
              }
              frame #1 {
              }
            }
          }
          frame #4 {
            n154 = property on="Y Step PV" class="DigNum (strict)"() -> ("Value"=w555:i32)  [unwired: 2 in, 2 out]
            n155 = property on="Y Step PV" class="DigNum (strict)"() -> ("Value"=w557:i32)  [unwired: 2 in, 2 out]
            n156 = property on="Y steps/rev" class="DigNum (strict)"() -> ("Value"=w559:u32)  [unwired: 2 in, 2 out]
            n157 = To Double Precision Float(number=w559) -> (double precision float=w553:dbl)
            n158 = property on="Y Step SP" class="DigNum (strict)"() -> ("Maximum"=w564:dbl)  [unwired: 2 in, 2 out]
            n159 = property on="Y Step SP" class="DigNum (strict)"() -> ("Minimum"=w565:dbl)  [unwired: 2 in, 2 out]
            n160 = To Double Precision Float(number=w555) -> (double precision float=w554:dbl)
            n161 = To Double Precision Float(number=w557) -> (double precision float=w556:dbl)
            n162 = Subtract(x=w565, y=w554) -> (x-y=w566:dbl)
            n163 = Subtract(x=w564, y=w556) -> (x-y=w563:dbl)
            n164 = property on="Y Scan Length SP steps" class="DigNum (strict)"() -> ("Value"=w561:i32)  [unwired: 2 in, 2 out]
            n165 = property on="Y Scan Velocity SP steps/sec" class="DigNum (strict)"() -> ("Value"=w552:i32)  [unwired: 2 in, 2 out]
            n166 = To Double Precision Float(number=w561) -> (double precision float=w560:dbl)
            n167 = property on="Y Scan Length SP steps" class="DigNum (strict)"("Minimum"=w566) -> ()  [unwired: 2 in, 2 out]
            n168 = property on="Y Scan Length SP steps" class="DigNum (strict)"("Maximum"=w563) -> ()  [unwired: 2 in, 2 out]
            n169 = Divide(x=w560, y=w553) -> (x/y=w562:dbl)
            n170 = To Double Precision Float(number=w552) -> (double precision float=w551:dbl)
            n171 = property on="Y mm/rev" class="DigNum (strict)"() -> ("Value"=w558:dbl)  [unwired: 2 in, 2 out]
            n172 = Multiply(x=w562, y=w558) -> (x*y=w549:dbl)
            n173 = Divide(x=w551, y=w553) -> (x/y=w550:dbl)
            n174 = Multiply(x=w558, y=w550) -> (x*y=w548:dbl)
            n175 = property on="Y Scan length MV mm" class="DigNum (strict)"("Value"=w549) -> ()  [unwired: 2 in, 2 out]
            n176 = property on="Y Scan velocity MV mm/sec" class="DigNum (strict)"("Val(Sgnl)"=w548) -> ()  [unwired: 2 in, 2 out]
          }
        }
        n177 = flat-sequence {
          tunnel: [w308] -> w255
          tunnel: [w284] -> w254
          tunnel: [w297] -> w253
          tunnel: [w275] -> w252
          tunnel: w242 -> [w274]
          tunnel: w241 -> [w273]
          tunnel: w255 -> [w314]
          tunnel: [w314] -> w251
          tunnel: w254 -> [w313]
          tunnel: [w313] -> w250
          tunnel: w253 -> [w312]
          tunnel: [w312] -> w249
          tunnel: w252 -> [w309]
          tunnel: [w309] -> w248
          tunnel: w251 -> [w321]
          tunnel: [w322] -> w247
          tunnel: w250 -> [w324]
          tunnel: [w323] -> w246
          tunnel: w249 -> [w320]
          tunnel: [w319] -> w245
          tunnel: w248 -> [w319]
          tunnel: w247 -> [w334]
          tunnel: w246 -> [w335]
          tunnel: [w333] -> w244
          tunnel: w245 -> [w337]
          tunnel: [w332] -> w243
          tunnel: [w420] -> w239
          tunnel: w244 -> [w420]
          tunnel: w243 -> [w400]
          tunnel: [w400] -> w240
          frame #0 {
            w279 = 0.1 ("Delay Time (s)")
            n178 = property on="X Step SP" class="DigNum (strict)"() -> ("Maximum"=w299:dbl)  [unwired: 2 in, 2 out]
            n179 = property on="X Step SP" class="DigNum (strict)"() -> ("Minimum"=w301:dbl)  [unwired: 2 in, 2 out]
            n180 = property on="X steps/rev" class="DigNum (strict)"() -> ("Value"=w295:u32)  [unwired: 2 in, 2 out]
            n181 = property on="X offset mm" class="DigNum (strict)"() -> ("Value"=w291:dbl)  [unwired: 2 in, 2 out]
            n182 = call "mDrive Send Command.vi"("error in (no error)"=w273, "Extra"="P", "Command"=T2."Print Parameter", "VISA resource name"=w274) -> ("error out"=w303:errorcluster, "read buffer"=w307:string, "VISA resource name out"=w305:refnum<visa-resource-name>)  [unwired: 3 in]
            n183 = call "Time Delay12"("error in (no error)"=w303, "Delay Time (s)"=w279) -> ("error out"=w302:errorcluster)  [unwired: 9 in]
            n184 = Decimal String To Number(string=w307, offset=0) -> (number=w287:i32)  [unwired: 1 in, 1 out]
            n185 = To Long Integer(number=w287) -> (32bit integer=w289:i32)
            n186 = property on="X Step PV" class="DigNum (strict)"("Val(Sgnl)"=w289) -> ()  [unwired: 2 in, 2 out]
            n187 = To Long Integer(number=w299) -> (32bit integer=w298:i32)
            n188 = To Long Integer(number=w301) -> (32bit integer=w300:i32)
            n189 = call "mDrive Send Command.vi"("error in (no error)"=w302, "Extra"="MV", "Command"=T2."Print Parameter", "VISA resource name"=w305) -> ("error out"=w304:errorcluster, "read buffer"=w285:string, "VISA resource name out"=w308:refnum<visa-resource-name>)  [unwired: 3 in]
            n190 = call "Time Delay11"("error in (no error)"=w304, "Delay Time (s)"=w279) -> ("error out"=w284:errorcluster)  [unwired: 9 in]
            n191 = In Range and Coerce(upper limit=w298, x=w289, lower limit=w300) -> (In Range?=w297:bool)  [unwired: 1 out]
            n192 = To Double Precision Float(number=w289) -> (double precision float=w290:dbl)
            n193 = To Double Precision Float(number=w295) -> (double precision float=w296:dbl)
            n194 = Decimal String To Number(string=w285, offset=0 ("offset (0)")) -> (number=w278:i32)  [unwired: 1 in, 1 out]
            n195 = property on="X  in Range" class="Bool (strict)"("Val(Sgnl)"=w297) -> ()  [unwired: 2 in, 2 out]
            n196 = Divide(x=w290, y=w296) -> (x/y=w294:dbl)
            n197 = Number To Boolean Array(number=w278) -> (Boolean array=w277:bool[])
            n198 = property on="X mm/rev" class="DigNum (strict)"() -> ("Value"=w293:dbl)  [unwired: 2 in, 2 out]
            n199 = Index Array(array=w277, index=0) -> (element=w275:bool)
            n200 = property on="X  in Motion" class="Bool (strict)"("Val(Sgnl)"=w275) -> ()  [unwired: 2 in, 2 out]
            n201 = Multiply(x=w294, y=w293) -> (x*y=w292:dbl)
            n202 = Add(x=w292, y=w291) -> (x+y=w288:dbl)
            n203 = property on="X Position mm PV" class="DigNum (strict)"("Val(Sgnl)"=w288) -> ()  [unwired: 2 in, 2 out]
          }
          frame #1 {
            n204 = property on="X Scan" class="Bool (strict)"() -> ("Value"=w310:bool)  [unwired: 2 in, 2 out]
            n205 = Or(x=w309, y=w310) -> (x .or. y?=w311:bool)
            n206 = case shown="False" w311 {
              frame #0 {
                n207 = property on="X Go" class="Bool"("DisabledEnum"=T1."Enabled" ("Disabled")) -> ()  [unwired: 2 in, 2 out]
                n208 = property on="X Scan OK" class="Bool"("DisabledEnum"=T1."Enabled" ("Disabled")) -> ()  [unwired: 2 in, 2 out]
              }
              frame #1 {
                n209 = property on="X Go" class="Bool"("DisabledEnum"=T1."Disabled and Grayed Out" ("Disabled")) -> ()  [unwired: 2 in, 2 out]
                n210 = property on="X Scan set" class="Bool"("DisabledEnum"=T1."Disabled and Grayed Out" ("Disabled")) -> ()  [unwired: 2 in, 2 out]
              }
            }
          }
          frame #2 {
            n211 = case shown="False" w320 {
              tunnel: w321 -> [w327 w331]
              tunnel: [w328 w331] -> w322
              tunnel: [w329 w330] -> w323
              tunnel: w324 -> [w326 w330]
              frame #0 {
                n212 = call "mDrive Send Command.vi"("error in (no error)"=w326, "Command"=T2."Stop", "VISA resource name"=w327) -> ("error out"=w329:errorcluster, "VISA resource name out"=w328:refnum<visa-resource-name>)  [unwired: 4 in, 1 out]
              }
              frame #1 {
              }
            }
          }
          frame #3 {
            n213 = property on="X Backlash corr" class="Bool (strict)"() -> ("Value"=w338:bool)  [unwired: 2 in, 2 out]
            n214 = Implies(1:w337, 2:w338) -> (0:w336:bool)
            n215 = case shown="False" w336 {
              tunnel: w335 -> [w345 w398]
              tunnel: w334 -> [w344 w399]
              tunnel: [w343 w398] -> w333
              tunnel: [w342 w399] -> w332
              frame #0 {
                # "Backlash"
                n216 = flat-sequence {
                  tunnel: [w360] -> w357
                  tunnel: [w362] -> w356
                  tunnel: [w361] -> w355
                  tunnel: w345 -> [w359]
                  tunnel: w344 -> [w358]
                  tunnel: w357 -> [w370]
                  tunnel: [w370] -> w354
                  tunnel: w356 -> [w369]
                  tunnel: w355 -> [w368]
                  tunnel: [w367] -> w353
                  tunnel: [w366] -> w352
                  tunnel: [w365] -> w341
                  tunnel: w354 -> [w380]
                  tunnel: w353 -> [w379]
                  tunnel: w352 -> [w377]
                  tunnel: [w378] -> w351
                  tunnel: [w377] -> w350
                  tunnel: [w376] -> w347
                  tunnel: [w375] -> w346
                  tunnel: w341 -> [w375]
                  tunnel: w351 -> [w391]
                  tunnel: w350 -> [w384]
                  tunnel: [w391] -> w349
                  tunnel: [w390] -> w348
                  tunnel: w347 -> [w390]
                  tunnel: w346 -> [w386]
                  tunnel: [w385] -> w339
                  tunnel: w349 -> [w395]
                  tunnel: w348 -> [w394]
                  tunnel: [w393] -> w343
                  tunnel: [w392] -> w340
                  tunnel: w339 -> [w392]
                  tunnel: [w397] -> w342
                  tunnel: w340 -> [w397]
                  frame #0 {
                    n217 = property on="X Backlash steps/sec" class="DigNum (strict)"() -> ("Value"=w360:i32)  [unwired: 2 in, 2 out]
                    n218 = Number To Decimal String(number=w360) -> (decimal integer string=w363:string)  [unwired: 1 in]
                    n219 = call "mDrive Send Command.vi"("error in (no error)"=w359, "Extra"=w363, "Command"=T2."Max Velocity", "VISA resource name"=w358) -> ("error out"=w361:errorcluster, "VISA resource name out"=w362:refnum<visa-resource-name>)  [unwired: 3 in, 1 out]
                  }
                  frame #1 {
                    n220 = property on="X Backlash" class="DigNum (strict)"() -> ("Value"=w365:i32)  [unwired: 2 in, 2 out]
                    n221 = Number To Decimal String(number=w365) -> (decimal integer string=w371:string)  [unwired: 1 in]
                    n222 = call "mDrive Send Command.vi"("error in (no error)"=w368, "Extra"=w371, "Command"=T2."Move to Relative Position", "VISA resource name"=w369) -> ("error out"=w367:errorcluster, "VISA resource name out"=w366:refnum<visa-resource-name>)  [unwired: 3 in, 1 out]
                  }
                  frame #2 {
                    n223 = To Double Precision Float(number=w375) -> (double precision float=w373:dbl)
                    n224 = To Double Precision Float(number=w380) -> (double precision float=w382:dbl)
                    n225 = Absolute Value(x=w373) -> (abs(x)=w374:dbl)
                    n226 = Divide(x=w374, y=w382) -> (x/y=w383:dbl)
                    n227 = Add(x=w383, y=0.3) -> (x+y=w376:dbl)
                    n228 = call "Time Delay13"("error in (no error)"=w379, "Delay Time (s)"=w376) -> ("error out"=w378:errorcluster)  [unwired: 9 in]
                  }
                  frame #3 {
                    n229 = Negate(x=w386) -> (-x=w387:i32)
                    n230 = Number To Decimal String(number=w387) -> (decimal integer string=w388:string)  [unwired: 1 in]
                    n231 = call "mDrive Send Command.vi"("Extra"=w388, "Command"=T2."Move to Relative Position", "VISA resource name"=w384) -> ("VISA resource name out"=w385:refnum<visa-resource-name>)  [unwired: 4 in, 2 out]
                  }
                  frame #4 {
                    n232 = call "Time Delay14"("error in (no error)"=w395, "Delay Time (s)"=w394) -> ("error out"=w393:errorcluster)  [unwired: 9 in]
                  }
                  frame #5 {
                    n233 = property on="X Backlash corr" class="Bool (strict)"("Val(Sgnl)"=FALSE ("Value (Signaling)")) -> ()  [unwired: 2 in, 2 out]
                  }
                }
              }
              frame #1 {
              }
            }
          }
          frame #4 {
            n234 = property on="X Step PV" class="DigNum (strict)"() -> ("Value"=w410:i32)  [unwired: 2 in, 2 out]
            n235 = property on="X Step PV" class="DigNum (strict)"() -> ("Value"=w408:i32)  [unwired: 2 in, 2 out]
            n236 = property on="X steps/rev" class="DigNum (strict)"() -> ("Value"=w412:u32)  [unwired: 2 in, 2 out]
            n237 = To Double Precision Float(number=w412) -> (double precision float=w406:dbl)
            n238 = property on="X Step SP" class="DigNum (strict)"() -> ("Maximum"=w417:dbl)  [unwired: 2 in, 2 out]
            n239 = property on="X Step SP" class="DigNum (strict)"() -> ("Minimum"=w418:dbl)  [unwired: 2 in, 2 out]
            n240 = To Double Precision Float(number=w408) -> (double precision float=w407:dbl)
            n241 = To Double Precision Float(number=w410) -> (double precision float=w409:dbl)
            n242 = Subtract(x=w417, y=w409) -> (x-y=w416:dbl)
            n243 = Subtract(x=w418, y=w407) -> (x-y=w419:dbl)
            n244 = property on="X Scan Length SP steps" class="DigNum (strict)"() -> ("Value"=w405:i32)  [unwired: 2 in, 2 out]
            n245 = property on="X Scan Velocity SP steps/sec" class="DigNum (strict)"() -> ("Value"=w414:i32)  [unwired: 2 in, 2 out]
            n246 = To Double Precision Float(number=w405) -> (double precision float=w404:dbl)
            n247 = property on="X Scan Length SP steps" class="DigNum (strict)"("Maximum"=w416) -> ()  [unwired: 2 in, 2 out]
            n248 = property on="X Scan Length SP steps" class="DigNum (strict)"("Minimum"=w419) -> ()  [unwired: 2 in, 2 out]
            n249 = Divide(x=w404, y=w406) -> (x/y=w403:dbl)
            n250 = To Double Precision Float(number=w414) -> (double precision float=w413:dbl)
            n251 = property on="X mm/rev" class="DigNum (strict)"() -> ("Value"=w411:dbl)  [unwired: 2 in, 2 out]
            n252 = Divide(x=w413, y=w406) -> (x/y=w415:dbl)
            n253 = Multiply(x=w411, y=w403) -> (x*y=w401:dbl)
            n254 = Multiply(x=w415, y=w411) -> (x*y=w402:dbl)
            n255 = property on="X Scan length MV mm" class="DigNum (strict)"("Val(Sgnl)"=w401) -> ()  [unwired: 2 in, 2 out]
            n256 = property on="X Scan velocity MV mm/sec" class="DigNum (strict)"("Value"=w402) -> ()  [unwired: 2 in, 2 out]
          }
        }
      }
      event #1 {
        n257 = event-data() -> ()  [unwired: 1 in, 5 out]
        n258 = property on="X Step SP" class="DigNum (strict)"() -> ("Value"=w573:i32)  [unwired: 2 in, 2 out]
        n259 = property on="X steps/rev" class="DigNum (strict)"() -> ("Value"=w571:u32)  [unwired: 2 in, 2 out]
        n260 = property on="X offset mm" class="DigNum (strict)"() -> ("Value"=w569:dbl)  [unwired: 2 in, 2 out]
        n261 = To Double Precision Float(number=w573) -> (double precision float=w574:dbl)
        n262 = To Double Precision Float(number=w571) -> (double precision float=w577:dbl)
        n263 = Divide(x=w574, y=w577) -> (x/y=w576:dbl)
        n264 = property on="X mm/rev" class="DigNum (strict)"() -> ("Value"=w570:dbl)  [unwired: 2 in, 2 out]
        n265 = Multiply(x=w576, y=w570) -> (x*y=w575:dbl)
        n266 = Add(x=w575, y=w569) -> (x+y=w572:dbl)
        n267 = property on="X Position MV mm" class="DigNum (strict)"("Val(Sgnl)"=w572) -> ()  [unwired: 2 in, 2 out]
      }
      event #2 {
        n268 = event-data() -> ()  [unwired: 1 in, 5 out]
        n269 = property on="Y steps/rev" class="DigNum (strict)"() -> ("Value"=w580:u32)  [unwired: 2 in, 2 out]
        n270 = property on="Y offset mm" class="DigNum (strict)"() -> ("Value"=w578:dbl)  [unwired: 2 in, 2 out]
        n271 = property on="Reset Y Position mm" class="DigNum (strict)"() -> ("Value"=w586:dbl)  [unwired: 2 in, 2 out]
        n272 = Subtract(x=w586, y=w578) -> (x-y=w585:dbl)
        n273 = property on="Y mm/rev" class="DigNum (strict)"() -> ("Value"=w579:dbl)  [unwired: 2 in, 2 out]
        n274 = Divide(x=w585, y=w579) -> (x/y=w584:dbl)
        n275 = To Double Precision Float(number=w580) -> (double precision float=w583:dbl)
        n276 = Multiply(x=w584, y=w583) -> (x*y=w582:dbl)
        n277 = To Long Integer(number=w582) -> (32bit integer=w581:i32)
        n278 = property on="Reset Y Motor Steps" class="DigNum (strict)"("Val(Sgnl)"=w581) -> ()  [unwired: 2 in, 2 out]
      }
      event #3 {
        n279 = event-data() -> ()  [unwired: 1 in, 5 out]
        n280 = property on="Y Step SP" class="DigNum (strict)"() -> ("Value"=w591:i32)  [unwired: 2 in, 2 out]
        n281 = property on="Y steps/rev" class="DigNum (strict)"() -> ("Value"=w589:u32)  [unwired: 2 in, 2 out]
        n282 = property on="Y offset mm" class="DigNum (strict)"() -> ("Value"=w587:dbl)  [unwired: 2 in, 2 out]
        n283 = To Double Precision Float(number=w591) -> (double precision float=w592:dbl)
        n284 = To Double Precision Float(number=w589) -> (double precision float=w595:dbl)
        n285 = Divide(x=w592, y=w595) -> (x/y=w594:dbl)
        n286 = property on="Y mm/rev" class="DigNum (strict)"() -> ("Value"=w588:dbl)  [unwired: 2 in, 2 out]
        n287 = Multiply(x=w594, y=w588) -> (x*y=w593:dbl)
        n288 = Add(x=w593, y=w587) -> (x+y=w590:dbl)
        n289 = property on="Y Position MV mm" class="DigNum (strict)"("Val(Sgnl)"=w590) -> ()  [unwired: 2 in, 2 out]
      }
      event #4 {
        n290 = event-data() -> ()  [unwired: 1 in, 5 out]
        n291 = property on="X Step SP" class="DigNum (strict)"() -> ("Value"=w600:i32)  [unwired: 2 in, 2 out]
        n292 = property on="X steps/rev" class="DigNum (strict)"() -> ("Value"=w598:u32)  [unwired: 2 in, 2 out]
        n293 = property on="X offset mm" class="DigNum (strict)"() -> ("Value"=w596:dbl)  [unwired: 2 in, 2 out]
        n294 = To Double Precision Float(number=w600) -> (double precision float=w601:dbl)
        n295 = To Double Precision Float(number=w598) -> (double precision float=w604:dbl)
        n296 = Divide(x=w601, y=w604) -> (x/y=w603:dbl)
        n297 = property on="X mm/rev" class="DigNum (strict)"() -> ("Value"=w597:dbl)  [unwired: 2 in, 2 out]
        n298 = Multiply(x=w603, y=w597) -> (x*y=w602:dbl)
        n299 = Add(x=w602, y=w596) -> (x+y=w599:dbl)
        n300 = property on="X Position MV mm" class="DigNum (strict)"("Val(Sgnl)"=w599) -> ()  [unwired: 2 in, 2 out]
      }
      event #5 {
        n301 = event-data() -> ()  [unwired: 1 in, 5 out]
        n302 = property on="Y steps/rev" class="DigNum (strict)"() -> ("Value"=w606:u32)  [unwired: 2 in, 2 out]
        n303 = property on="Y Velocity SP step/sec" class="DigNum (strict)"() -> ("Value"=w608:i32)  [unwired: 2 in, 2 out]
        n304 = To Double Precision Float(number=w608) -> (double precision float=w609:dbl)
        n305 = To Double Precision Float(number=w606) -> (double precision float=w611:dbl)
        n306 = Divide(x=w609, y=w611) -> (x/y=w610:dbl)
        n307 = property on="Y mm/rev" class="DigNum (strict)"() -> ("Value"=w605:dbl)  [unwired: 2 in, 2 out]
        n308 = Multiply(x=w610, y=w605) -> (x*y=w607:dbl)
        n309 = property on="Y Velocity MV mm/sec" class="DigNum (strict)"("Val(Sgnl)"=w607) -> ()  [unwired: 2 in, 2 out]
      }
      event #6 {
        n310 = event-data() -> ()  [unwired: 1 in, 5 out]
        n311 = property on="X steps/rev" class="DigNum (strict)"() -> ("Value"=w613:u32)  [unwired: 2 in, 2 out]
        n312 = property on="X Velocity SP step/sec" class="DigNum (strict)"() -> ("Value"=w615:i32)  [unwired: 2 in, 2 out]
        n313 = To Double Precision Float(number=w615) -> (double precision float=w616:dbl)
        n314 = To Double Precision Float(number=w613) -> (double precision float=w618:dbl)
        n315 = Divide(x=w616, y=w618) -> (x/y=w617:dbl)
        n316 = property on="X mm/rev" class="DigNum (strict)"() -> ("Value"=w612:dbl)  [unwired: 2 in, 2 out]
        n317 = Multiply(x=w617, y=w612) -> (x*y=w614:dbl)
        n318 = property on="X Velocity MV mm/sec" class="DigNum (strict)"("Val(Sgnl)"=w614) -> ()  [unwired: 2 in, 2 out]
      }
      event #7 {
        n319 = event-data() -> ()  [unwired: 1 in, 7 out]
        n320 = flat-sequence {
          frame #0 {
            n321 = property on="Y steps/rev" class="DigNum (strict)"() -> ("Value"=w626:u32)  [unwired: 2 in, 2 out]
            n322 = property on="Y offset mm" class="DigNum (strict)"() -> ("Value"=w624:dbl)  [unwired: 2 in, 2 out]
            n323 = property on="Y Position SP mm" class="DigNum (strict)"() -> ("Value"=w623:dbl)  [unwired: 2 in, 2 out]
            n324 = Subtract(x=w623, y=w624) -> (x-y=w628:dbl)
            n325 = property on="Y mm/rev" class="DigNum (strict)"() -> ("Value"=w627:dbl)  [unwired: 2 in, 2 out]
            n326 = Divide(x=w628, y=w627) -> (x/y=w629:dbl)
            n327 = To Double Precision Float(number=w626) -> (double precision float=w630:dbl)
            n328 = Multiply(x=w629, y=w630) -> (x*y=w622:dbl)
            n329 = property on="Y Step SP" class="DigNum (strict)"() -> ("Maximum"=w620:dbl)  [unwired: 2 in, 2 out]
            n330 = property on="Y Step SP" class="DigNum (strict)"() -> ("Minimum"=w619:dbl)  [unwired: 2 in, 2 out]
            n331 = In Range and Coerce(upper limit=w620, x=w622, lower limit=w619) -> (coerced(x)=w621:dbl)  [unwired: 1 out]
            n332 = To Long Integer(number=w621) -> (32bit integer=w625:i32)
            n333 = property on="Y Step SP" class="DigNum (strict)"("Val(Sgnl)"=w625) -> ()  [unwired: 2 in, 2 out]
          }
          frame #1 {
            n334 = property on="Y steps/rev" class="DigNum (strict)"() -> ("Value"=w636:u32)  [unwired: 2 in, 2 out]
            n335 = To Double Precision Float(number=w636) -> (double precision float=w637:dbl)
            n336 = property on="Y Velocity SP step/sec" class="DigNum (strict)"() -> ("Maximum"=w632:dbl)  [unwired: 2 in, 2 out]
            n337 = property on="Y Velocity SP step/sec" class="DigNum (strict)"() -> ("Minimum"=w631:dbl)  [unwired: 2 in, 2 out]
            n338 = property on="Y Velocity SP mm/sec" class="DigNum (strict)"() -> ("Value"=w638:dbl)  [unwired: 2 in, 2 out]
            n339 = property on="Y mm/rev" class="DigNum (strict)"() -> ("Value"=w640:dbl)  [unwired: 2 in, 2 out]
            n340 = Divide(x=w638, y=w640) -> (x/y=w639:dbl)
            n341 = Multiply(x=w639, y=w637) -> (x*y=w634:dbl)
            n342 = In Range and Coerce(upper limit=w632, x=w634, lower limit=w631) -> (coerced(x)=w633:dbl)  [unwired: 1 out]
            n343 = To Long Integer(number=w633) -> (32bit integer=w635:i32)
            n344 = property on="Y Velocity SP step/sec" class="DigNum (strict)"("Val(Sgnl)"=w635) -> ()  [unwired: 2 in, 2 out]
          }
        }
      }
      event #8 {
        n345 = event-data() -> ()  [unwired: 1 in, 7 out]
        n346 = flat-sequence {
          frame #0 {
            n347 = property on="X steps/rev" class="DigNum (strict)"() -> ("Value"=w648:u32)  [unwired: 2 in, 2 out]
            n348 = property on="X offset mm" class="DigNum (strict)"() -> ("Value"=w646:dbl)  [unwired: 2 in, 2 out]
            n349 = property on="X Position SP mm" class="DigNum (strict)"() -> ("Value"=w645:dbl)  [unwired: 2 in, 2 out]
            n350 = Subtract(x=w645, y=w646) -> (x-y=w650:dbl)
            n351 = property on="X mm/rev" class="DigNum (strict)"() -> ("Value"=w649:dbl)  [unwired: 2 in, 2 out]
            n352 = Divide(x=w650, y=w649) -> (x/y=w651:dbl)
            n353 = To Double Precision Float(number=w648) -> (double precision float=w652:dbl)
            n354 = Multiply(x=w651, y=w652) -> (x*y=w644:dbl)
            n355 = property on="X Step SP" class="DigNum (strict)"() -> ("Maximum"=w642:dbl)  [unwired: 2 in, 2 out]
            n356 = property on="X Step SP" class="DigNum (strict)"() -> ("Minimum"=w641:dbl)  [unwired: 2 in, 2 out]
            n357 = In Range and Coerce(upper limit=w642, x=w644, lower limit=w641) -> (coerced(x)=w643:dbl)  [unwired: 1 out]
            n358 = To Long Integer(number=w643) -> (32bit integer=w647:i32)
            n359 = property on="X Step SP" class="DigNum (strict)"("Val(Sgnl)"=w647) -> ()  [unwired: 2 in, 2 out]
          }
          frame #1 {
            n360 = property on="X steps/rev" class="DigNum (strict)"() -> ("Value"=w658:u32)  [unwired: 2 in, 2 out]
            n361 = To Double Precision Float(number=w658) -> (double precision float=w659:dbl)
            n362 = property on="X Velocity SP step/sec" class="DigNum (strict)"() -> ("Maximum"=w654:dbl)  [unwired: 2 in, 2 out]
            n363 = property on="X Velocity SP step/sec" class="DigNum (strict)"() -> ("Minimum"=w653:dbl)  [unwired: 2 in, 2 out]
            n364 = property on="X Scan Velocity SP mm/sec" class="DigNum (strict)"() -> ("Value"=w660:dbl)  [unwired: 2 in, 2 out]
            n365 = property on="X mm/rev" class="DigNum (strict)"() -> ("Value"=w662:dbl)  [unwired: 2 in, 2 out]
            n366 = Divide(x=w660, y=w662) -> (x/y=w661:dbl)
            n367 = Multiply(x=w661, y=w659) -> (x*y=w656:dbl)
            n368 = In Range and Coerce(upper limit=w654, x=w656, lower limit=w653) -> (coerced(x)=w655:dbl)  [unwired: 1 out]
            n369 = To Long Integer(number=w655) -> (32bit integer=w657:i32)
            n370 = property on="X Velocity SP step/sec" class="DigNum (strict)"("Val(Sgnl)"=w657) -> ()  [unwired: 2 in, 2 out]
          }
        }
      }
      event #9 {
        n371 = event-data() -> ()  [unwired: 1 in, 7 out]
        n372 = flat-sequence {
          frame #0 {
            n373 = property on="Y steps/rev" class="DigNum (strict)"() -> ("Value"=w669:u32)  [unwired: 2 in, 2 out]
            n374 = To Double Precision Float(number=w669) -> (double precision float=w672:dbl)
            n375 = property on="Y Scan Length SP mm" class="DigNum (strict)"() -> ("Value"=w667:dbl)  [unwired: 2 in, 2 out]
            n376 = property on="Y mm/rev" class="DigNum (strict)"() -> ("Value"=w670:dbl)  [unwired: 2 in, 2 out]
            n377 = Divide(x=w667, y=w670) -> (x/y=w671:dbl)
            n378 = Multiply(x=w671, y=w672) -> (x*y=w666:dbl)
            n379 = property on="Y Step SP" class="DigNum (strict)"() -> ("Maximum"=w663:dbl)  [unwired: 2 in, 2 out]
            n380 = property on="Y Step SP" class="DigNum (strict)"() -> ("Minimum"=w664:dbl)  [unwired: 2 in, 2 out]
            n381 = In Range and Coerce(upper limit=w663, x=w666, lower limit=w664) -> (coerced(x)=w665:dbl)  [unwired: 1 out]
            n382 = To Long Integer(number=w665) -> (32bit integer=w668:i32)
            n383 = property on="Y Scan Length SP steps" class="DigNum (strict)"("Val(Sgnl)"=w668) -> ()  [unwired: 2 in, 2 out]
          }
          frame #1 {
            n384 = property on="Y steps/rev" class="DigNum (strict)"() -> ("Value"=w678:u32)  [unwired: 2 in, 2 out]
            n385 = To Double Precision Float(number=w678) -> (double precision float=w679:dbl)
            n386 = property on="Y Scan Velocity SP mm/sec" class="DigNum (strict)"() -> ("Value"=w680:dbl)  [unwired: 2 in, 2 out]
            n387 = property on="Y Scan Velocity SP steps/sec" class="DigNum (strict)"() -> ("Maximum"=w674:dbl)  [unwired: 2 in, 2 out]
            n388 = property on="Y Scan Velocity SP steps/sec" class="DigNum (strict)"() -> ("Minimum"=w673:dbl)  [unwired: 2 in, 2 out]
            n389 = property on="Y mm/rev" class="DigNum (strict)"() -> ("Value"=w682:dbl)  [unwired: 2 in, 2 out]
            n390 = Divide(x=w680, y=w682) -> (x/y=w681:dbl)
            n391 = Multiply(x=w681, y=w679) -> (x*y=w676:dbl)
            n392 = In Range and Coerce(upper limit=w674, x=w676, lower limit=w673) -> (coerced(x)=w675:dbl)  [unwired: 1 out]
            n393 = To Long Integer(number=w675) -> (32bit integer=w677:i32)
            n394 = property on="Y Scan Velocity SP steps/sec" class="DigNum (strict)"("Val(Sgnl)"=w677) -> ()  [unwired: 2 in, 2 out]
          }
        }
      }
      event #10 {
        n395 = event-data() -> ()  [unwired: 1 in, 7 out]
        n396 = flat-sequence {
          frame #0 {
            n397 = property on="X steps/rev" class="DigNum (strict)"() -> ("Value"=w689:u32)  [unwired: 2 in, 2 out]
            n398 = To Double Precision Float(number=w689) -> (double precision float=w692:dbl)
            n399 = property on="X Scan Length SP mm" class="DigNum (strict)"() -> ("Value"=w687:dbl)  [unwired: 2 in, 2 out]
            n400 = property on="X mm/rev" class="DigNum (strict)"() -> ("Value"=w690:dbl)  [unwired: 2 in, 2 out]
            n401 = Divide(x=w687, y=w690) -> (x/y=w691:dbl)
            n402 = Multiply(x=w691, y=w692) -> (x*y=w686:dbl)
            n403 = property on="X Step SP" class="DigNum (strict)"() -> ("Maximum"=w683:dbl)  [unwired: 2 in, 2 out]
            n404 = property on="X Step SP" class="DigNum (strict)"() -> ("Minimum"=w684:dbl)  [unwired: 2 in, 2 out]
            n405 = In Range and Coerce(upper limit=w683, x=w686, lower limit=w684) -> (coerced(x)=w685:dbl)  [unwired: 1 out]
            n406 = To Long Integer(number=w685) -> (32bit integer=w688:i32)
            n407 = property on="X Scan Length SP steps" class="DigNum (strict)"("Val(Sgnl)"=w688) -> ()  [unwired: 2 in, 2 out]
          }
          frame #1 {
            n408 = property on="X steps/rev" class="DigNum (strict)"() -> ("Value"=w698:u32)  [unwired: 2 in, 2 out]
            n409 = To Double Precision Float(number=w698) -> (double precision float=w699:dbl)
            n410 = property on="X Scan Velocity SP mm/sec" class="DigNum (strict)"() -> ("Value"=w700:dbl)  [unwired: 2 in, 2 out]
            n411 = property on="X Scan Velocity SP steps/sec" class="DigNum (strict)"() -> ("Maximum"=w694:dbl)  [unwired: 2 in, 2 out]
            n412 = property on="X Scan Velocity SP steps/sec" class="DigNum (strict)"() -> ("Minimum"=w693:dbl)  [unwired: 2 in, 2 out]
            n413 = property on="X mm/rev" class="DigNum (strict)"() -> ("Value"=w702:dbl)  [unwired: 2 in, 2 out]
            n414 = Divide(x=w700, y=w702) -> (x/y=w701:dbl)
            n415 = Multiply(x=w701, y=w699) -> (x*y=w696:dbl)
            n416 = In Range and Coerce(upper limit=w694, x=w696, lower limit=w693) -> (coerced(x)=w695:dbl)  [unwired: 1 out]
            n417 = To Long Integer(number=w695) -> (32bit integer=w697:i32)
            n418 = property on="X Scan Velocity SP steps/sec" class="DigNum (strict)"("Val(Sgnl)"=w697) -> ()  [unwired: 2 in, 2 out]
          }
        }
      }
      event #11 {
        n419 = event-data() -> ()  [unwired: 1 in, 7 out]
        n420 = flat-sequence {
          tunnel: w707 -> [w717]
          tunnel: w708 -> [w718]
          tunnel: [w718] -> w704
          tunnel: [w717] -> w703
          tunnel: [w721] -> w706
          tunnel: [w720] -> w705
          tunnel: w704 -> [w723]
          tunnel: w703 -> [w722]
          tunnel: [w741] -> w710
          tunnel: [w740] -> w709
          tunnel: w706 -> [w739]
          tunnel: w705 -> [w738]
          tunnel: [w748] -> w712
          tunnel: [w747] -> w711
          tunnel: w710 -> [w746]
          tunnel: w709 -> [w745]
          tunnel: [w754] -> w713
          tunnel: [w755] -> w714
          tunnel: w712 -> [w755]
          tunnel: w711 -> [w753]
          frame #0 {
            n421 = property on="Y Go" class="Bool"("DisabledEnum"=T1."Disabled and Grayed Out" ("Disabled")) -> ()  [unwired: 2 in, 2 out]
            n422 = property on="Scan Go" class="Bool"("DisabledEnum"=T1."Disabled and Grayed Out" ("Disabled")) -> ()  [unwired: 2 in, 2 out]
          }
          frame #1 {
            n423 = property on="Y Step SP" class="DigNum (strict)"() -> ("Value"=w731:i32)  [unwired: 2 in, 2 out]
            n424 = property on="Y Step PV" class="DigNum (strict)"() -> ("Value"=w730:i32)  [unwired: 2 in, 2 out]
            n425 = property on="Y Backlash" class="DigNum (strict)"() -> ("Value"=w719:i32)  [unwired: 2 in, 2 out]
            n426 = Subtract(x=w731, y=w730) -> (x-y=w729:i32)
            n427 = Sign(1:w719) -> (0:w727:i32)
            n428 = Sign(1:w729) -> (0:w728:i32)
            n429 = Multiply(x=w728, y=w727) -> (x*y=w726:i32)
            n430 = Equal?(x=w726, y=1) -> (x = y?=w724:bool)
            n431 = case shown="False" w724 {
              tunnel: w723 -> [w734 w736]
              tunnel: w722 -> [w733 w735]
              tunnel: [w733 w735] -> w721
              tunnel: [w734 w736] -> w720
              frame #0 {
                n432 = property on="Y Backlash corr" class="Bool (strict)"("Val(Sgnl)"=FALSE ("Value (Signaling)")) -> ()  [unwired: 2 in, 2 out]
              }
              frame #1 {
                n433 = property on="Y Backlash corr" class="Bool (strict)"("Val(Sgnl)"=TRUE ("Value (Signaling)")) -> ()  [unwired: 2 in, 2 out]
              }
            }
          }
          frame #2 {
            # "Velocity Setting"
            n434 = property on="Y Velocity SP step/sec" class="DigNum (strict)"() -> ("Value"=w742:i32)  [unwired: 2 in, 2 out]
            n435 = Number To Decimal String(number=w742) -> (decimal integer string=w743:string)  [unwired: 1 in]
            n436 = call "mDrive Send Command.vi"("error in (no error)"=w739, "Extra"=w743, "Command"=T2."Max Velocity", "VISA resource name"=w738) -> ("error out"=w740:errorcluster, "VISA resource name out"=w741:refnum<visa-resource-name>)  [unwired: 3 in, 1 out]
          }
          frame #3 {
            # "Move to Abs Position"
            n437 = property on="Y Step SP" class="DigNum (strict)"() -> ("Value"=w751:i32)  [unwired: 2 in, 2 out]
            n438 = Number To Decimal String(number=w751) -> (decimal integer string=w750:string)  [unwired: 1 in]
            n439 = call "mDrive Send Command.vi"("error in (no error)"=w745, "Extra"=w750, "Command"=T2."Move to Absolute Position", "VISA resource name"=w746) -> ("error out"=w747:errorcluster, "VISA resource name out"=w748:refnum<visa-resource-name>)  [unwired: 3 in, 1 out]
          }
          frame #4 {
            n440 = call "Time Delay"("error in (no error)"=w753, "Delay Time (s)"=0.1) -> ("error out"=w754:errorcluster)  [unwired: 9 in]
          }
        }
      }
      event #12 {
        n441 = event-data() -> ()  [unwired: 1 in, 7 out]
        n442 = flat-sequence {
          tunnel: [w769] -> w761
          tunnel: [w768] -> w760
          tunnel: w759 -> [w769]
          tunnel: w758 -> [w768]
          tunnel: [w774] -> w763
          tunnel: [w773] -> w762
          tunnel: w761 -> [w776]
          tunnel: w760 -> [w775]
          tunnel: [w794] -> w765
          tunnel: [w793] -> w764
          tunnel: w763 -> [w792]
          tunnel: w762 -> [w791]
          tunnel: [w801] -> w767
          tunnel: [w800] -> w766
          tunnel: w765 -> [w799]
          tunnel: w764 -> [w798]
          tunnel: [w807] -> w756
          tunnel: [w808] -> w757
          tunnel: w767 -> [w808]
          tunnel: w766 -> [w806]
          frame #0 {
            n443 = property on="X Go" class="Bool"("DisabledEnum"=T1."Disabled and Grayed Out" ("Disabled")) -> ()  [unwired: 2 in, 2 out]
            n444 = property on="Scan Go" class="Bool"("DisabledEnum"=T1."Disabled and Grayed Out" ("Disabled")) -> ()  [unwired: 2 in, 2 out]
          }
          frame #1 {
            n445 = property on="X Step SP" class="DigNum (strict)"() -> ("Value"=w784:i32)  [unwired: 2 in, 2 out]
            n446 = property on="X Step PV" class="DigNum (strict)"() -> ("Value"=w783:i32)  [unwired: 2 in, 2 out]
            n447 = property on="X Backlash" class="DigNum (strict)"() -> ("Value"=w772:i32)  [unwired: 2 in, 2 out]
            n448 = Subtract(x=w784, y=w783) -> (x-y=w782:i32)
            n449 = Sign(1:w772) -> (0:w780:i32)
            n450 = Sign(1:w782) -> (0:w781:i32)
            n451 = Multiply(x=w781, y=w780) -> (x*y=w779:i32)
            n452 = Equal?(x=w779, y=1) -> (x = y?=w777:bool)
            n453 = case shown="False" w777 {
              tunnel: w776 -> [w787 w789]
              tunnel: w775 -> [w786 w788]
              tunnel: [w786 w788] -> w774
              tunnel: [w787 w789] -> w773
              frame #0 {
                n454 = property on="X Backlash corr" class="Bool (strict)"("Val(Sgnl)"=FALSE ("Value (Signaling)")) -> ()  [unwired: 2 in, 2 out]
              }
              frame #1 {
                n455 = property on="Y Backlash corr" class="Bool (strict)"("Val(Sgnl)"=TRUE ("Value (Signaling)")) -> ()  [unwired: 2 in, 2 out]
              }
            }
          }
          frame #2 {
            # "Velocity Setting"
            n456 = property on="X Scan Velocity SP steps/sec" class="DigNum (strict)"() -> ("Value"=w795:i32)  [unwired: 2 in, 2 out]
            n457 = Number To Decimal String(number=w795) -> (decimal integer string=w796:string)  [unwired: 1 in]
            n458 = call "mDrive Send Command.vi"("error in (no error)"=w792, "Extra"=w796, "Command"=T2."Max Velocity", "VISA resource name"=w791) -> ("error out"=w793:errorcluster, "VISA resource name out"=w794:refnum<visa-resource-name>)  [unwired: 3 in, 1 out]
          }
          frame #3 {
            # "Move to Abs Position"
            n459 = property on="X Step SP" class="DigNum (strict)"() -> ("Value"=w804:i32)  [unwired: 2 in, 2 out]
            n460 = Number To Decimal String(number=w804) -> (decimal integer string=w803:string)  [unwired: 1 in]
            n461 = call "mDrive Send Command.vi"("error in (no error)"=w798, "Extra"=w803, "Command"=T2."Move to Absolute Position", "VISA resource name"=w799) -> ("error out"=w800:errorcluster, "VISA resource name out"=w801:refnum<visa-resource-name>)  [unwired: 3 in, 1 out]
          }
          frame #4 {
            n462 = call "Time Delay15"("error in (no error)"=w806, "Delay Time (s)"=0.1) -> ("error out"=w807:errorcluster)  [unwired: 9 in]
          }
        }
      }
      event #13 {
        n463 = event-data() -> ()  [unwired: 1 in, 7 out]
        n464 = flat-sequence {
          tunnel: [w824] -> w816
          tunnel: [w822] -> w815
          tunnel: w814 -> [w818]
          tunnel: w813 -> [w817]
          tunnel: w816 -> [w839]
          tunnel: w815 -> [w838]
          tunnel: [w839] -> w810
          tunnel: [w838] -> w809
          tunnel: [w842] -> w811
          tunnel: [w843] -> w812
          tunnel: w810 -> [w843]
          tunnel: w809 -> [w842]
          frame #0 {
            # "VELOCITY"
            n465 = property on="X Scan Velocity SP steps/sec" class="DigNum (strict)"() -> ("Value"=w825:i32)  [unwired: 2 in, 2 out]
            n466 = Number To Decimal String(number=w825) -> (decimal integer string=w826:string)  [unwired: 1 in]
            n467 = call "mDrive Send Command.vi"("error in (no error)"=w817, "Extra"=w826, "Command"=T2."Max Velocity", "VISA resource name"=w818) -> ("error out"=w827:errorcluster, "VISA resource name out"=w832:refnum<visa-resource-name>)  [unwired: 3 in, 1 out]
            n468 = call "Time Delay9"("error in (no error)"=w827) -> ("error out"=w830:errorcluster)  [unwired: 10 in]
            n469 = call "mDrive Send Command.vi"("error in (no error)"=w830, "Extra"="VM", "Command"=T2."Print Parameter", "VISA resource name"=w832) -> ("error out"=w823:errorcluster, "read buffer"=w828:string, "VISA resource name out"=w824:refnum<visa-resource-name>)  [unwired: 3 in]
            n470 = call "Time Delay10"("error in (no error)"=w823) -> ("error out"=w822:errorcluster)  [unwired: 10 in]
            n471 = Decimal String To Number(string=w828, offset=0) -> (number=w831:i32)  [unwired: 1 in, 1 out]
            n472 = property on="X scan steps/sec MV step/sec" class="DigNum (strict)"("Val(Sgnl)"=w831) -> ()  [unwired: 2 in, 2 out]
          }
          frame #1 {
            n473 = property on="X Scan" class="Bool (strict)"("Val(Sgnl)"=TRUE ("Slew Ready 2")) -> ()  [unwired: 2 in, 2 out]
            n474 = property on="Scan Go" class="Bool"("DisabledEnum"=T1."Enabled" ("Disabled")) -> ()  [unwired: 2 in, 2 out]
            n475 = property on="Scan Cancel" class="Bool"("DisabledEnum"=T1."Enabled" ("Disabled")) -> ()  [unwired: 2 in, 2 out]
            n476 = property on="X Scan Velocity SP steps/sec" class="DigNum (strict)"("DisabledEnum"=T1."Disabled and Grayed Out" ("Disabled")) -> ()  [unwired: 2 in, 2 out]
            n477 = property on="X Scan Length SP steps" class="DigNum (strict)"("DisabledEnum"=T1."Disabled and Grayed Out" ("Disabled")) -> ()  [unwired: 2 in, 2 out]
          }
          frame #2 {
            n478 = property on="X Go" class="Bool"("DisabledEnum"=T1."Disabled and Grayed Out" ("Disabled")) -> ()  [unwired: 2 in, 2 out]
            n479 = property on="Y Go" class="Bool"("DisabledEnum"=T1."Disabled and Grayed Out" ("Disabled")) -> ()  [unwired: 2 in, 2 out]
          }
        }
      }
      event #14 {
        n480 = event-data() -> ()  [unwired: 1 in, 7 out]
        n481 = flat-sequence {
          tunnel: w851 -> [w861]
          tunnel: w850 -> [w860]
          tunnel: [w857] -> w848
          tunnel: [w855] -> w847
          tunnel: w848 -> [w874]
          tunnel: w847 -> [w873]
          tunnel: [w874] -> w845
          tunnel: [w873] -> w844
          tunnel: [w877] -> w849
          tunnel: [w878] -> w846
          tunnel: w845 -> [w878]
          tunnel: w844 -> [w877]
          frame #0 {
            # "VELOCITY"
            n482 = property on="Y Scan Velocity SP steps/sec" class="DigNum (strict)"() -> ("Value"=w858:i32)  [unwired: 2 in, 2 out]
            n483 = Number To Decimal String(number=w858) -> (decimal integer string=w859:string)  [unwired: 1 in]
            n484 = call "mDrive Send Command.vi"("error in (no error)"=w861, "Extra"=w859, "Command"=T2."Max Velocity", "VISA resource name"=w860) -> ("error out"=w862:errorcluster, "VISA resource name out"=w867:refnum<visa-resource-name>)  [unwired: 3 in, 1 out]
            n485 = call "Time Delay5"("error in (no error)"=w862) -> ("error out"=w865:errorcluster)  [unwired: 10 in]
            n486 = call "mDrive Send Command.vi"("error in (no error)"=w865, "Extra"="VM", "Command"=T2."Print Parameter", "VISA resource name"=w867) -> ("error out"=w856:errorcluster, "read buffer"=w863:string, "VISA resource name out"=w857:refnum<visa-resource-name>)  [unwired: 3 in]
            n487 = call "Time Delay6"("error in (no error)"=w856) -> ("error out"=w855:errorcluster)  [unwired: 10 in]
            n488 = Decimal String To Number(string=w863, offset=0) -> (number=w866:i32)  [unwired: 1 in, 1 out]
            n489 = property on="Y scan steps/sec MV step/sec" class="DigNum (strict)"("Val(Sgnl)"=w866) -> ()  [unwired: 2 in, 2 out]
          }
          frame #1 {
            n490 = property on="Y Scan" class="Bool (strict)"("Val(Sgnl)"=TRUE ("Slew Ready 2")) -> ()  [unwired: 2 in, 2 out]
            n491 = property on="Scan Go" class="Bool"("DisabledEnum"=T1."Enabled" ("Disabled")) -> ()  [unwired: 2 in, 2 out]
            n492 = property on="Scan Cancel" class="Bool"("DisabledEnum"=T1."Enabled" ("Disabled")) -> ()  [unwired: 2 in, 2 out]
            n493 = property on="Y Scan Velocity SP steps/sec" class="DigNum (strict)"("DisabledEnum"=T1."Disabled and Grayed Out" ("Disabled")) -> ()  [unwired: 2 in, 2 out]
            n494 = property on="Y Scan Length SP steps" class="DigNum (strict)"("DisabledEnum"=T1."Disabled and Grayed Out" ("Disabled")) -> ()  [unwired: 2 in, 2 out]
          }
          frame #2 {
            n495 = property on="X Go" class="Bool"("DisabledEnum"=T1."Disabled and Grayed Out" ("Disabled")) -> ()  [unwired: 2 in, 2 out]
            n496 = property on="Y Go" class="Bool"("DisabledEnum"=T1."Disabled and Grayed Out" ("Disabled")) -> ()  [unwired: 2 in, 2 out]
          }
        }
      }
      event #15 {
        n497 = event-data() -> ()  [unwired: 1 in, 4 out]
        n498 = event-data() -> ()  [unwired: 3 in, 1 out]
      }
      event #16 {
        n499 = event-data() -> ()  [unwired: 1 in, 7 out]
        n500 = call "mDrive Send Command.vi"("error in (no error)"=w890, "Command"=T2."Stop", "VISA resource name"=w891) -> ("error out"=w888:errorcluster, "VISA resource name out"=w889:refnum<visa-resource-name>)  [unwired: 4 in, 1 out]
        n501 = call "mDrive Send Command.vi"("error in (no error)"=w882, "Command"=T2."Stop", "VISA resource name"=w883) -> ("error out"=w884:errorcluster, "VISA resource name out"=w885:refnum<visa-resource-name>)  [unwired: 4 in, 1 out]
      }
      event #17 {
        n502 = event-data() -> ()  [unwired: 1 in, 7 out]
        n503 = flat-sequence {
          tunnel: w903 -> [w921]
          tunnel: w902 -> [w920]
          tunnel: [w923] -> w899
          tunnel: [w922] -> w898
          tunnel: [w930] -> w904
          tunnel: [w931] -> w905
          tunnel: w899 -> [w931]
          tunnel: w898 -> [w930]
          frame #0 {
            n504 = call "mDrive Send Command.vi"("error in (no error)"=w920, "Command"=T2."Stop", "VISA resource name"=w921) -> ("error out"=w922:errorcluster, "VISA resource name out"=w923:refnum<visa-resource-name>)  [unwired: 4 in, 1 out]
          }
          frame #1 {
            n505 = property on="Y Scan" class="Bool (strict)"("Value"=FALSE ("Slew Ready")) -> ()  [unwired: 2 in, 2 out]
            n506 = property on="Y Scan OK" class="Bool"("DisabledEnum"=T1."Enabled" ("Disabled")) -> ()  [unwired: 2 in, 2 out]
            n507 = property on="Y Scan Length SP steps" class="DigNum (strict)"("DisabledEnum"=T1."Enabled" ("Disabled")) -> ()  [unwired: 2 in, 2 out]
            n508 = property on="Y Scan OK" class="Bool"("DisabledEnum"=T1."Enabled" ("Disabled")) -> ()  [unwired: 2 in, 2 out]
            n509 = property on="Y Scan Velocity SP steps/sec" class="DigNum (strict)"("DisabledEnum"=T1."Enabled" ("Disabled")) -> ()  [unwired: 2 in, 2 out]
            n510 = property on="Y Go" class="Bool"("DisabledEnum"=T1."Enabled" ("Disabled")) -> ()  [unwired: 2 in, 2 out]
          }
        }
        n511 = flat-sequence {
          tunnel: w895 -> [w908]
          tunnel: w894 -> [w907]
          tunnel: [w910] -> w897
          tunnel: [w909] -> w896
          tunnel: [w917] -> w892
          tunnel: [w918] -> w893
          tunnel: w897 -> [w918]
          tunnel: w896 -> [w917]
          frame #0 {
            n512 = call "mDrive Send Command.vi"("error in (no error)"=w907, "Command"=T2."Stop", "VISA resource name"=w908) -> ("error out"=w909:errorcluster, "VISA resource name out"=w910:refnum<visa-resource-name>)  [unwired: 4 in, 1 out]
          }
          frame #1 {
            n513 = property on="X Scan" class="Bool (strict)"("Value"=FALSE ("Slew Ready")) -> ()  [unwired: 2 in, 2 out]
            n514 = property on="X Scan set" class="Bool"("DisabledEnum"=T1."Enabled" ("Disabled")) -> ()  [unwired: 2 in, 2 out]
            n515 = property on="X Scan Velocity SP steps/sec" class="DigNum (strict)"("DisabledEnum"=T1."Enabled" ("Disabled")) -> ()  [unwired: 2 in, 2 out]
            n516 = property on="X Scan Length SP steps" class="DigNum (strict)"("DisabledEnum"=T1."Enabled" ("Disabled")) -> ()  [unwired: 2 in, 2 out]
            n517 = property on="X Go" class="Bool"("DisabledEnum"=T1."Enabled" ("Disabled")) -> ()  [unwired: 2 in, 2 out]
            n518 = property on="X Scan OK" class="Bool"("DisabledEnum"=T1."Enabled" ("Disabled")) -> ()  [unwired: 2 in, 2 out]
          }
        }
        n519 = property on="Scan Go" class="Bool"("DisabledEnum"=T1."Disabled and Grayed Out" ("Disabled")) -> ()  [unwired: 2 in, 2 out]
        n520 = property on="Scan Cancel" class="Bool"("DisabledEnum"=T1."Disabled and Grayed Out" ("Disabled")) -> ()  [unwired: 2 in, 2 out]
      }
      event #18 {
        n521 = event-data() -> ()  [unwired: 1 in, 7 out]
        n522 = property on="Y Scan" class="Bool (strict)"() -> ("Value"=w935:bool)  [unwired: 2 in, 2 out]
        n523 = flat-sequence {
          tunnel: w948 -> [w951]
          tunnel: w947 -> [w952]
          tunnel: [w952] -> w944
          tunnel: [w951] -> w943
          tunnel: [w950] -> w942
          tunnel: w935 -> [w949]
          tunnel: [w949] -> w934
          tunnel: w944 -> [w963]
          tunnel: [w965] -> w939
          tunnel: w943 -> [w962]
          tunnel: [w964] -> w937
          tunnel: w942 -> [w961]
          tunnel: w934 -> [w960]
          tunnel: [w960] -> w932
          tunnel: w939 -> [w976]
          tunnel: [w976] -> w938
          tunnel: w937 -> [w975]
          tunnel: [w975] -> w936
          tunnel: [w973] -> w933
          tunnel: w932 -> [w973]
          tunnel: w938 -> [w981]
          tunnel: [w979] -> w941
          tunnel: w936 -> [w980]
          tunnel: [w978] -> w940
          tunnel: w933 -> [w977]
          tunnel: w941 -> [w997]
          tunnel: w940 -> [w996]
          tunnel: [w997] -> w946
          tunnel: [w996] -> w945
          frame #0 {
            n524 = case shown="True" w949 {
              tunnel: ["" w954] -> w950
              frame #0 {
              }
              frame #1 {
                n525 = property on="Y Scan Length SP steps" class="DigNum (strict)"() -> ("Value"=w959:i32)  [unwired: 2 in, 2 out]
                n526 = Number To Decimal String(number=w959) -> (decimal integer string=w956:string)  [unwired: 1 in]
                n527 = call <vilib>:"Space Constant.vi"() -> ("String"=w957:string)
                n528 = Concatenate Strings("MR", w957, w956, "\r") -> (w954:string)
              }
            }
          }
          frame #1 {
            n529 = case shown="True" w960 {
              tunnel: [w967 w972] -> w965
              tunnel: [w966 w971] -> w964
              tunnel: w963 -> [w967 w970]
              tunnel: w962 -> [w966 w969]
              tunnel: w961 -> [_ w968]
              frame #0 {
              }
              frame #1 {
                n530 = VISA Write(VISA resource name=w970, write buffer=w968, error in (no error)=w969) -> (VISA resource name out=w972:refnum<visa-resource-name>, error out=w971:errorcluster)  [unwired: 1 out]
              }
            }
          }
          frame #2 {
            n531 = call "Time Delay7"("Delay Time (s)"=0.1) -> ()  [unwired: 10 in, 1 out]
          }
          frame #3 {
            n532 = case shown="True" w977 {
              tunnel: w981 -> [w983 w987]
              tunnel: w980 -> [w982 w986]
              tunnel: [w983 w985] -> w979
              tunnel: [w982 w984] -> w978
              frame #0 {
              }
              frame #1 {
                n533 = property class="Instr"(reference=w987, error in=w986) -> (reference out=w989:refnum<visa-resource-name>, error out=w988:errorcluster, "Serial Settings:Number of Bytes at Serial Port"=w990:u32)
                n534 = VISA Read(VISA resource name=w989, byte count=w990, error in (no error)=w988) -> (VISA resource name out=w985:refnum<visa-resource-name>, error out=w984:errorcluster)  [unwired: 2 out]
              }
            }
          }
          frame #4 {
            n535 = property on="Y Scan" class="Bool (strict)"("Val(Sgnl)"=FALSE ("Slew Ready 2")) -> ()  [unwired: 2 in, 2 out]
            n536 = property on="Slew Velocity" class="DigNum (strict)"("DisabledEnum"=T1."Enabled" ("Disabled")) -> ()  [unwired: 2 in, 2 out]
            n537 = property on="Y Scan Length SP steps" class="DigNum (strict)"("DisabledEnum"=T1."Enabled" ("Disabled")) -> ()  [unwired: 2 in, 2 out]
            n538 = property on="Scan Go" class="Bool"("DisabledEnum"=T1."Disabled and Grayed Out" ("Disabled")) -> ()  [unwired: 2 in, 2 out]
            n539 = property on="Scan Cancel" class="Bool"("DisabledEnum"=T1."Disabled and Grayed Out" ("Disabled")) -> ()  [unwired: 2 in, 2 out]
          }
        }
      }
      event #19 {
        n540 = event-data() -> ()  [unwired: 1 in, 7 out]
        n541 = flat-sequence {
          tunnel: w1005 -> [w1016]
          tunnel: w1004 -> [w1015]
          tunnel: [w1014] -> w1003
          tunnel: [w1013] -> w1002
          frame #0 {
            n542 = property on="Reset Y Motor Steps" class="DigNum (strict)"() -> ("Value"=w1017:i32)  [unwired: 2 in, 2 out]
            n543 = Number To Decimal String(number=w1017) -> (decimal integer string=w1018:string)  [unwired: 1 in]
            n544 = call "mDrive Send Command.vi"("error in (no error)"=w1015, "Extra"=w1018, "Command"=T2."Set Current Position", "VISA resource name"=w1016) -> ("error out"=w1013:errorcluster, "VISA resource name out"=w1014:refnum<visa-resource-name>)  [unwired: 3 in, 1 out]
          }
        }
        n545 = flat-sequence {
          tunnel: [w1006] -> w999
          tunnel: w1000 -> [w1009]
          tunnel: [w1008] -> _
          tunnel: [w1007] -> w998
          tunnel: w1001 -> [w1006]
          frame #0 {
            n546 = property on="Reset X Motor Steps" class="DigNum (strict)"() -> ("Value"=w1010:i32)  [unwired: 2 in, 2 out]
            n547 = Number To Decimal String(number=w1010) -> (decimal integer string=w1011:string)  [unwired: 1 in]
            n548 = call "mDrive Send Command.vi"("error in (no error)"=w1009, "Extra"=w1011, "Command"=T2."Set Current Position", "VISA resource name"=w1006) -> ("error out"=w1007:errorcluster, "VISA resource name out"=w1008:refnum<visa-resource-name>)  [unwired: 3 in, 1 out]
          }
        }
      }
    }
    n549 = flat-sequence {
      frame #0 {
      }
    }
  }
  n550 = flat-sequence {
    tunnel: w55 -> [w1024]
    tunnel: w54 -> [w1021]
    frame #0 {
      n551 = call "mDrive Send Command.vi"("error in (no error)"=w1021, "Command"=T2."Stop", "VISA resource name"=w1024) -> ("error out"=w1022:errorcluster, "VISA resource name out"=w1023:refnum<visa-resource-name>)  [unwired: 4 in, 1 out]
      n552 = VISA Close(VISA resource name=w1023, error in (no error)=w1022) -> ()  [unwired: 1 out]
    }
  }
  n553 = flat-sequence {
    tunnel: w26 -> [w1029]
    tunnel: w25 -> [w1026]
    frame #0 {
      n554 = call "mDrive Send Command.vi"("error in (no error)"=w1026, "Command"=T2."Stop", "VISA resource name"=w1029) -> ("error out"=w1027:errorcluster, "VISA resource name out"=w1028:refnum<visa-resource-name>)  [unwired: 4 in, 1 out]
      n555 = VISA Close(VISA resource name=w1028, error in (no error)=w1027) -> ()  [unwired: 1 out]
    }
  }
  "Y COM PORT" <- w58
  "X COM PORT" <- w31
  "Z COM PORT" <- w18
